vi "AutoFocus.vi"(0 "Function":T23, 1 "Set Inverse Matrix":T4, 5 "Displacement":dbl(slide) scale=1.0..1000.0, 7 "Matching Criteria":T7={"Minimum Score"=700.0, "Color Score Weight"=700.0, "Minimum Contrast"=50, "Match Mode"=0, "Match Feature Mode"=0, "Subpixel Accuracy"=TRUE, "Color Sensitivity"=1, "Search Strategy"=1} {"Match Mode" items=["Shift Invariant", "Rotation Invariant"]; "Match Feature Mode" items=["Color and Shape", "Color", "Shape"]; "Color Sensitivity" items=["Low Sensitivity", "Medium Sensitivity", "High Sensitivity"]; "Search Strategy" items=["Conservative", "Balance", "Aggressive", "Very Aggressive"]}, 9 "Z Scan Parameters":T3={"Z Range"=1380.0, "Resolution"=5000.0, "Initial Direction"=enum."Up", "Focus Threshold"=0.1, "Ascent Constant"=0.1} {"Focus Threshold" min=0.0 max=1000.0 step=1.0 format="%#_2f"; "Ascent Constant" min=0.0 max=1000.0 step=1.0 format="%#_2f"; "Resolution" min=0.0 max=1.0 step=0.01 format="%_2g"; "Z Range" format="%_3g"}, 11 "error in (no error)":errorcluster, 12 "Refnums":T21, 13 "Notifiers":T8, 14 "Message Queues out":T6) -> (4 "Target Found?":bool, 6 "Transformation Matrix":T4, 8 "Target Data":T5, 15 "error out":errorcluster)   [LabVIEW 2014]
uses:
  AutoFocus Functions.ctl
  AutoFocus Refnums.ctl
  support/Instrument Status.ctl
  ZScan.ctl
  <vilib>/Analysis/Matrix/Datatypes/RealMatrix.ctl
  Target Refnums.ctl
  support/Notifiers/Notifiers.ctl
  support/Message Handler Loop Notifiers.ctl
  Parameter Analyzer/Parameter Analyzer Notifiers.ctl
  Switching Matrix/Switching Matrix Notifiers.ctl
  Stress Control/StressControl Notifiers.ctl
  Spectrometer/Spectrometer Notifiers.ctl
  Switches and Mirrors/SwitchesMirrors Notifiers.ctl
  Camera/Camera Notifiers.ctl
  XYZ Stage/XYZ Notifications.ctl
  Autofocus Notifiers.ctl
  Measurements/Optoelectronic Measurement/Optoelectronic Notifiers.ctl
  Measurements/Save Data/SaveData Notifiers.ctl
  Measurements/Instrument Sequence/Instrument Sequence Notifiers.ctl
  support/Message Queue/All Message Queues.ctl
  support/Message Queue/Message Cluster.ctl
  support/Instrument Status State.ctl
  Target Functions.ctl
  <vilib>/Analysis/baseanly.llb/Matrix Type of Inverse Matrix.ctl
  XYZ Stage/XYZ Config.ctl
  XYZ Stage/XYZ Connection Settings.ctl
  XYZ Stage/XYZ Stage Control.ctl
  XYZ Stage/XYZ Coordinate Control.ctl
  <vilib>/Analysis/baseanly.llb/A x Vector.vi
  <vilib>/Analysis/baseanly.llb/Real Inverse Matrix.vi
  support/Message Queue/Message Queue.lvlib
  <vilib>/Analysis/NI_AALBase.lvlib
  <vilib>/Analysis/Matrix/NI_Matrix.lvlib
panel:
  out "Edge Detection Array":T1
  out "Instrument Status":T2
  out "Matching Curves":cluster{dbl[], sgl[]}[](graph)
  # "LICENSED MATERIALS – PROPERTY OF IBM\nCopyright IBM Corp. 2016,\nALL RIGHTS RESERVED"
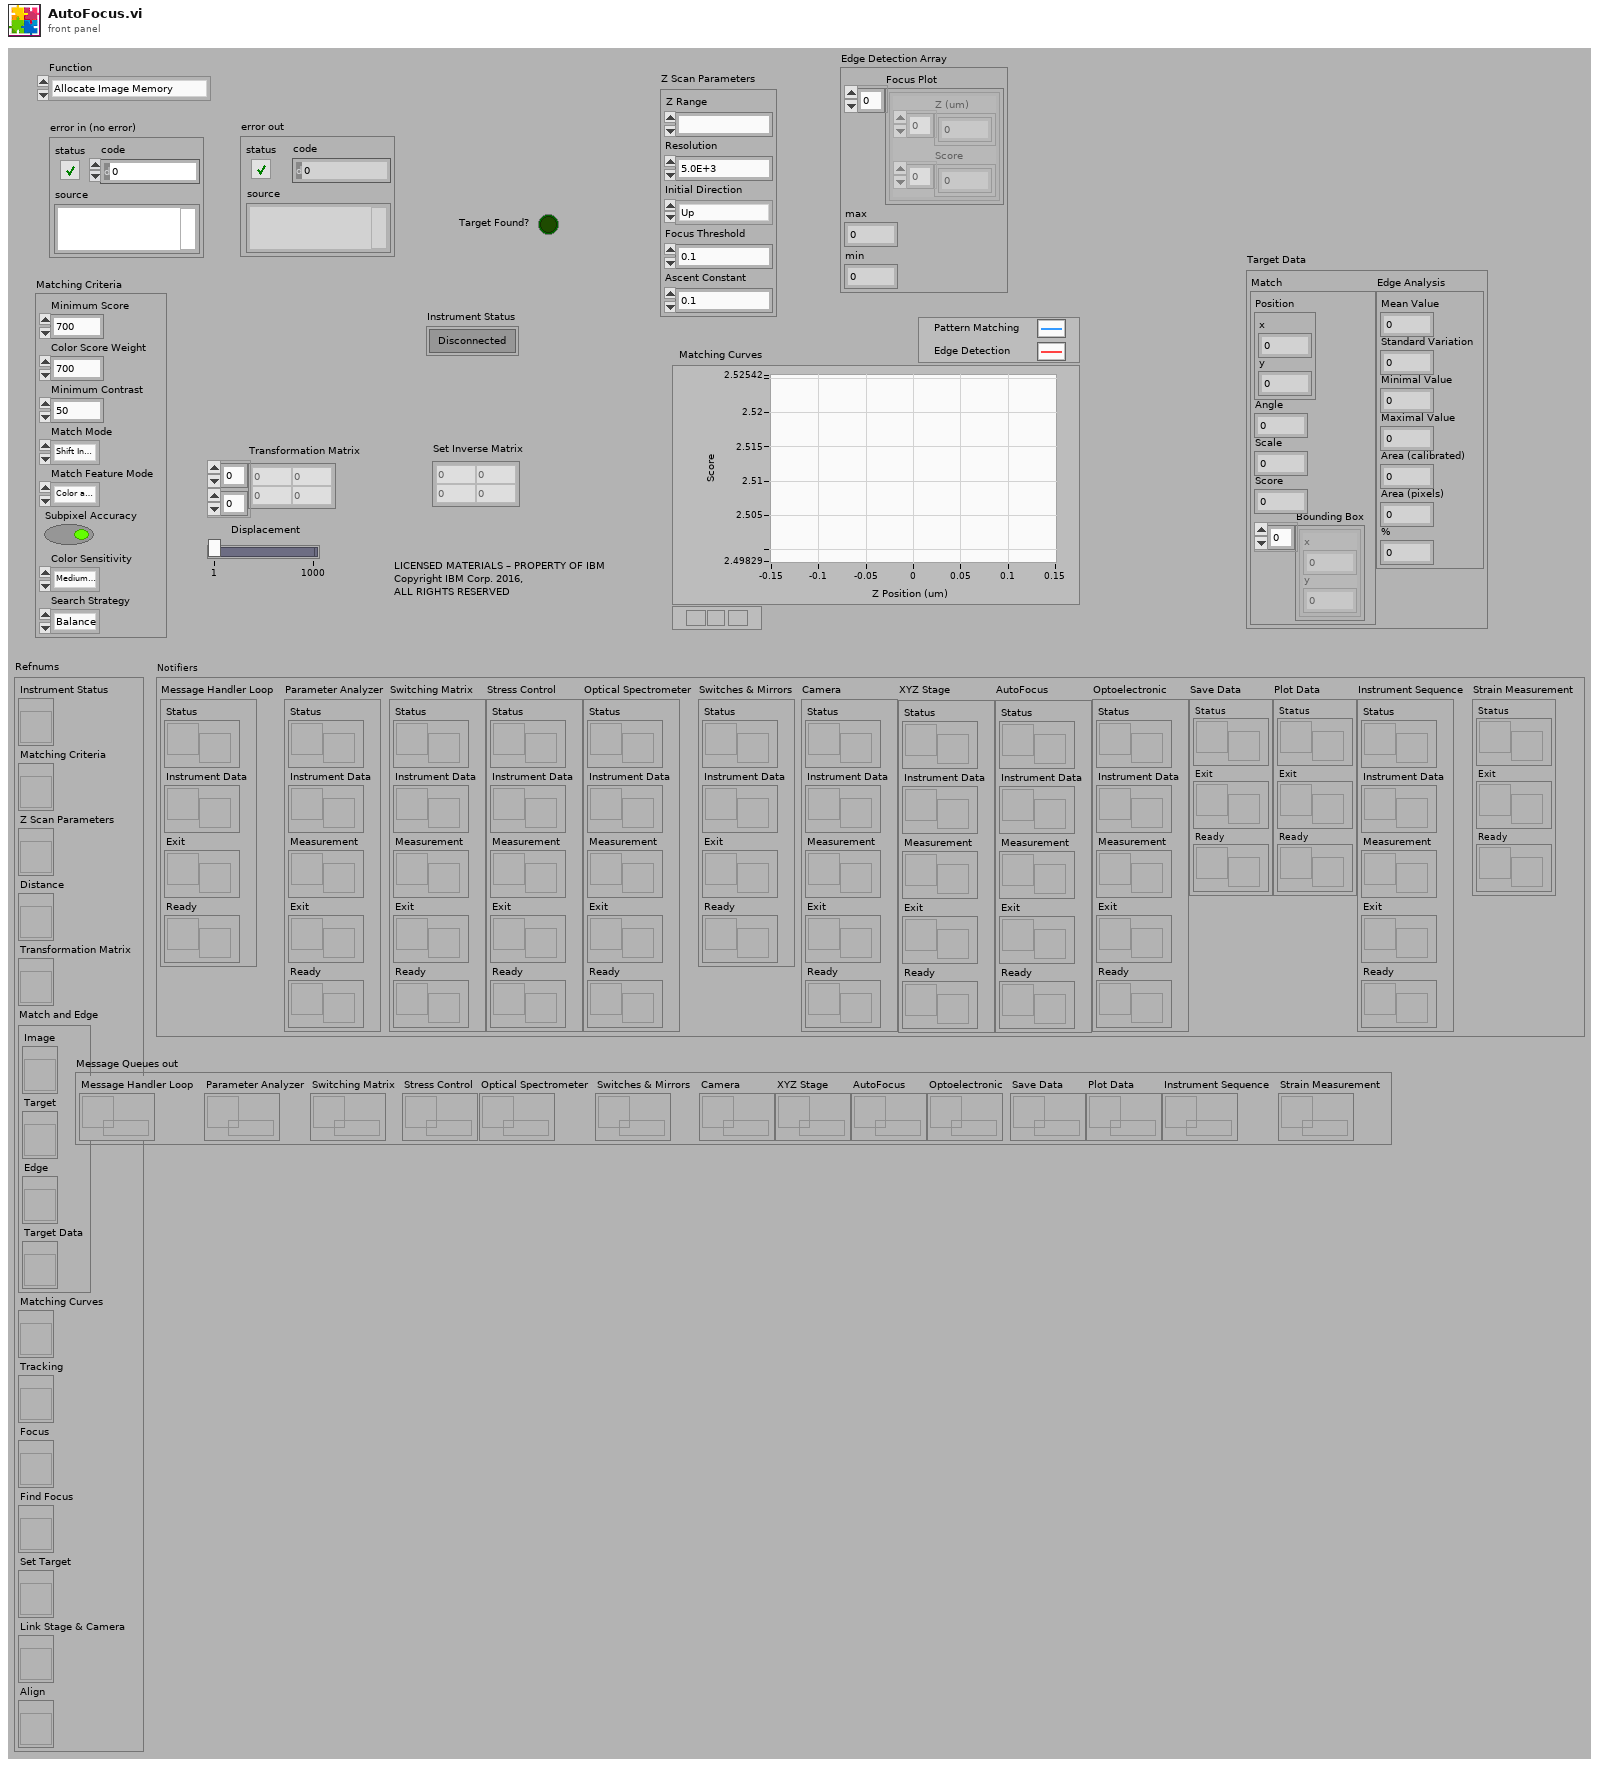
[diagram p1: front panel]
types:
  T1 = cluster{"Focus Plot":cluster{"Z (um)":dbl[], "Score":sgl[]}[], "max":sgl, "min":sgl}
  T2 = typedef "Instrument Status.ctl" = bool
  T3 = typedef "ZScan.ctl" = cluster{"Z Range":ext, "Resolution":dbl, "Initial Direction":enum16{"Up", "Down"}, "Focus Threshold":dbl, "Ascent Constant":dbl}
  T4 = typedef "NI_Matrix.lvlib/RealMatrix.ctl" = dbl[][]
  T5 = cluster{"Match":cluster{"Position":cluster{"x":sgl, "y":sgl}, "Angle":sgl, "Scale":sgl, "Score":sgl, "Bounding Box":cluster{"x":sgl, "y":sgl}[]}, "Edge Analysis":cluster{"Mean Value":sgl, "Standard Variation":sgl, "Minimal Value":sgl, "Maximal Value":sgl, "Area (calibrated)":sgl, "Area (pixels)":i32, "%":sgl}}
  T6 = typedef "Message Queue.lvlib/All Message Queues.ctl" = cluster{"Message Handler Loop":refnum<queue>, "Parameter Analyzer":refnum<queue>, "Switching Matrix":refnum<queue>, "Stress Control":refnum<queue>, "Optical Spectrometer":refnum<queue>, "Switches & Mirrors":refnum<queue>, "Camera":refnum<queue>, "XYZ Stage":refnum<queue>, "AutoFocus":refnum<queue>, "Optoelectronic":refnum<queue>, "Save Data":refnum<queue>, "Plot Data":refnum<queue>, "Instrument Sequence":refnum<queue>, "Strain Measurement":refnum<queue>}
  T7 = cluster{"Minimum Score":sgl, "Color Score Weight":sgl, "Minimum Contrast":i32, "Match Mode":u32, "Match Feature Mode":u32, "Subpixel Accuracy":bool, "Color Sensitivity":u32, "Search Strategy":u32}
  T8 = typedef "Notifiers.ctl" = cluster{"Message Handler Loop":T9, "Parameter Analyzer":T10, "Switching Matrix":T11, "Stress Control":T12, "Optical Spectrometer":T13, "Switches & Mirrors":T14, "Camera":T15, "XYZ Stage":T16, "AutoFocus":T17, "Optoelectronic":T18, "Save Data":T19, "Plot Data":T19, "Instrument Sequence":T20, "Strain Measurement":cluster{"Status":refnum<notifier>, "Exit":refnum<notifier>, "Ready":refnum<notifier>}}
  T9 = typedef "Message Handler Loop Notifiers.ctl" = cluster{"Status":refnum<notifier>, "Instrument Data":refnum<notifier>, "Exit":refnum<notifier>, "Ready":refnum<notifier>}
  T10 = typedef "Parameter Analyzer Notifiers.ctl" = cluster{"Status":refnum<notifier>, "Instrument Data":refnum<notifier>, "Measurement":refnum<notifier>, "Exit":refnum<notifier>, "Ready":refnum<notifier>}
  T11 = typedef "Switching Matrix Notifiers.ctl" = cluster{"Status":refnum<notifier>, "Instrument Data":refnum<notifier>, "Measurement":refnum<notifier>, "Exit":refnum<notifier>, "Ready":refnum<notifier>}
  T12 = typedef "StressControl Notifiers.ctl" = cluster{"Status":refnum<notifier>, "Instrument Data":refnum<notifier>, "Measurement":refnum<notifier>, "Exit":refnum<notifier>, "Ready":refnum<notifier>}
  T13 = typedef "Spectrometer Notifiers.ctl" = cluster{"Status":refnum<notifier>, "Instrument Data":refnum<notifier>, "Measurement":refnum<notifier>, "Exit":refnum<notifier>, "Ready":refnum<notifier>}
  T14 = typedef "SwitchesMirrors Notifiers.ctl" = cluster{"Status":refnum<notifier>, "Instrument Data":refnum<notifier>, "Exit":refnum<notifier>, "Ready":refnum<notifier>}
  T15 = typedef "Camera Notifiers.ctl" = cluster{"Status":refnum<notifier>, "Instrument Data":refnum<notifier>, "Measurement":refnum<notifier>, "Exit":refnum<notifier>, "Ready":refnum<notifier>}
  T16 = typedef "XYZ Notifications.ctl" = cluster{"Status":refnum<notifier>, "Instrument Data":refnum<notifier>, "Measurement":refnum<notifier>, "Exit":refnum<notifier>, "Ready":refnum<notifier>}
  T17 = typedef "Autofocus Notifiers.ctl" = cluster{"Status":refnum<notifier>, "Instrument Data":refnum<notifier>, "Measurement":refnum<notifier>, "Exit":refnum<notifier>, "Ready":refnum<notifier>}
  T18 = typedef "Optoelectronic Notifiers.ctl" = cluster{"Status":refnum<notifier>, "Instrument Data":refnum<notifier>, "Measurement":refnum<notifier>, "Exit":refnum<notifier>, "Ready":refnum<notifier>}
  T19 = typedef "SaveData Notifiers.ctl" = cluster{"Status":refnum<notifier>, "Exit":refnum<notifier>, "Ready":refnum<notifier>}
  T20 = typedef "Instrument Sequence Notifiers.ctl" = cluster{"Status":refnum<notifier>, "Instrument Data":refnum<notifier>, "Measurement":refnum<notifier>, "Exit":refnum<notifier>, "Ready":refnum<notifier>}
  T21 = typedef "AutoFocus Refnums.ctl" = cluster{"Instrument Status":refnum<vi>, "Matching Criteria":refnum<vi>, "Z Scan Parameters":refnum<vi>, "Distance":refnum<vi>, "Transformation Matrix":refnum<vi>, "Match and Edge":T22, "Matching Curves":refnum<vi>, "Tracking":refnum<vi>, "Focus":refnum<vi>, "Find Focus":refnum<vi>, "Set Target":refnum<vi>, "Link Stage & Camera":refnum<vi>, "Align":refnum<vi>}
  T22 = typedef "Target Refnums.ctl" = cluster{"Image":refnum<vi>, "Target":refnum<vi>, "Edge":refnum<vi>, "Target Data":refnum<vi>}
  T23 = typedef "AutoFocus Functions.ctl" = enum16{"Allocate Image Memory", "Free Image Memory", "Grab Image", "Get ROI", "Set ROI", "Set Match Criteria", "Set Target", "Link Stage & Camera", "Set Transformation Matrix", "Find Target", "Align", "Find Focus", "Focus (Gradient)", "Focus (Threshold)", "Focus (Turning Points)", "Update Refnums"}
  T24 = typedef "Instrument Status State.ctl" = enum16{"Unknown", "Idle", "Standby", "Configuring", "Measuring", "Moving", "Disconnected"}
  T25 = typedef "Image Type" = u32
  T26 = cluster{"Border Size":i32, "Image Name":string, "Image Type":T25}[]
  T27 = typedef "Target Functions.ctl" = enum16{"Setup Match Criteria", "Set Target", "Find Target"}
  T28 = typedef "NI_AALBase.lvlib/Matrix Type of Inverse Matrix.ctl" = enum32{"General", "Positive Definite", "Lower Triangular", "Upper Triangular"}
  T29 = typedef "XYZ Config.ctl" = cluster{"Connection Settings":T30, "Manual Control":T31, "Coordinate Control":T32}
  T30 = typedef "XYZ Connection Settings.ctl" = cluster{"Tango VISA":refnum<visa-resource-name>, "Baudrate":i32, "Show Protocol?":bool}
  T31 = typedef "XYZ Stage Control.ctl" = cluster{"North":bool, "South":bool, "West":bool, "East":bool, "Up":bool, "Down":bool, "Stop":bool, "XY Step":dbl, "Z step":dbl}
  T32 = typedef "XYZ Coordinate Control.ctl" = cluster{"Motion Mode":enum16{"Absolute", "Relative"}, "Destination [mm]":dbl[]}
  T33 = typedef "IMAQ Image.ctl" = refnum<image>
  T34 = cluster{"Global Rectangle":i32[], "Contours":cluster{"Contour Type":u32, "ROI Type":u32, "Points":i32[]}[]}
  T35 = cluster{"Registers Filled?":bool, "Negative Edge Slope?":bool, "Negative Z Slope?":bool, "Focus at Edge?":bool}
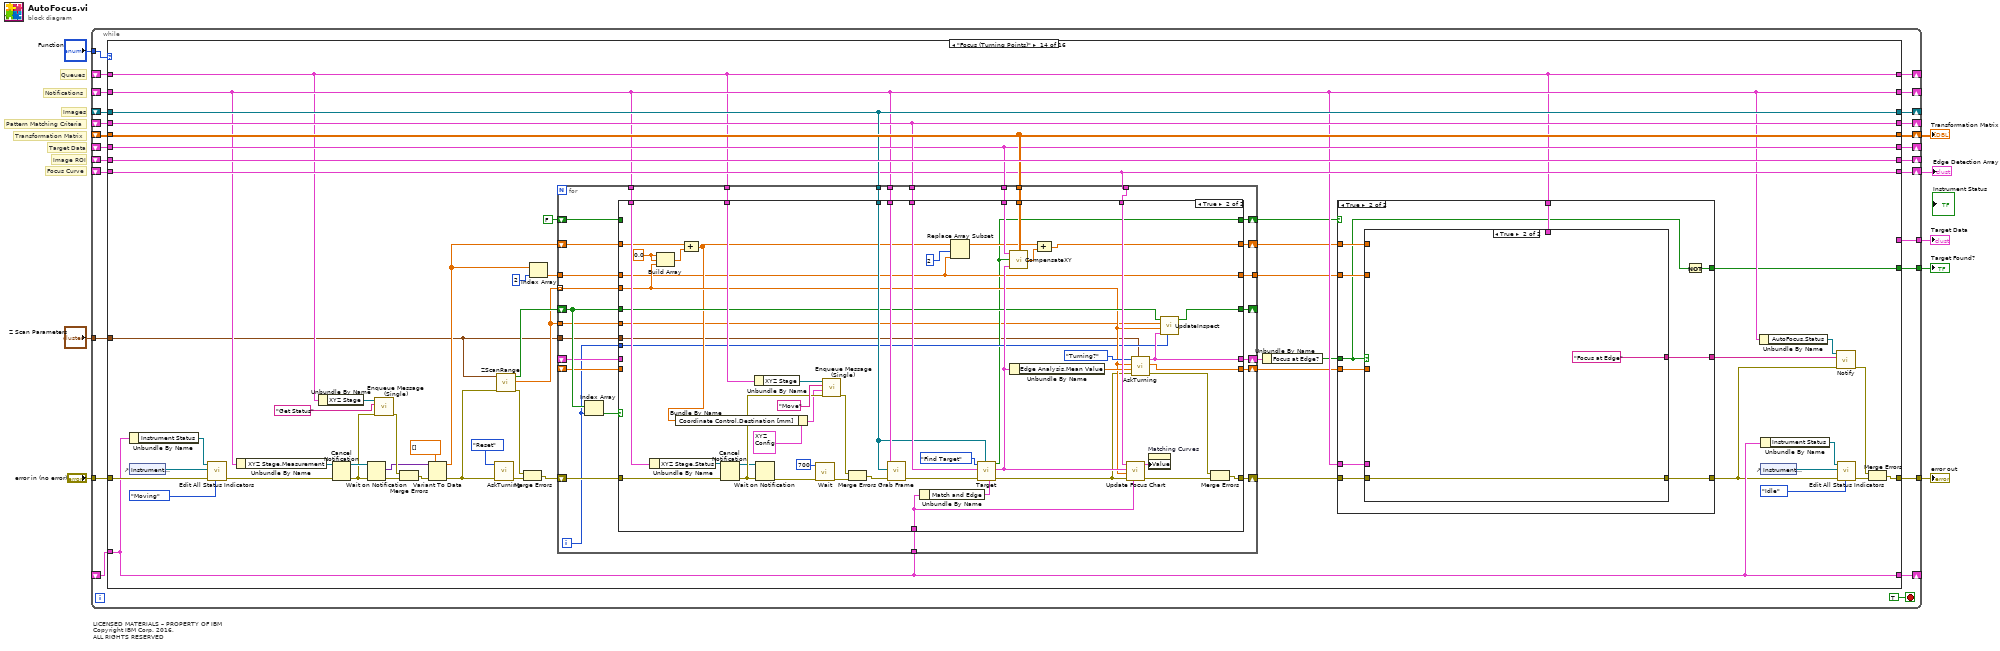
[diagram p0: block diagram]
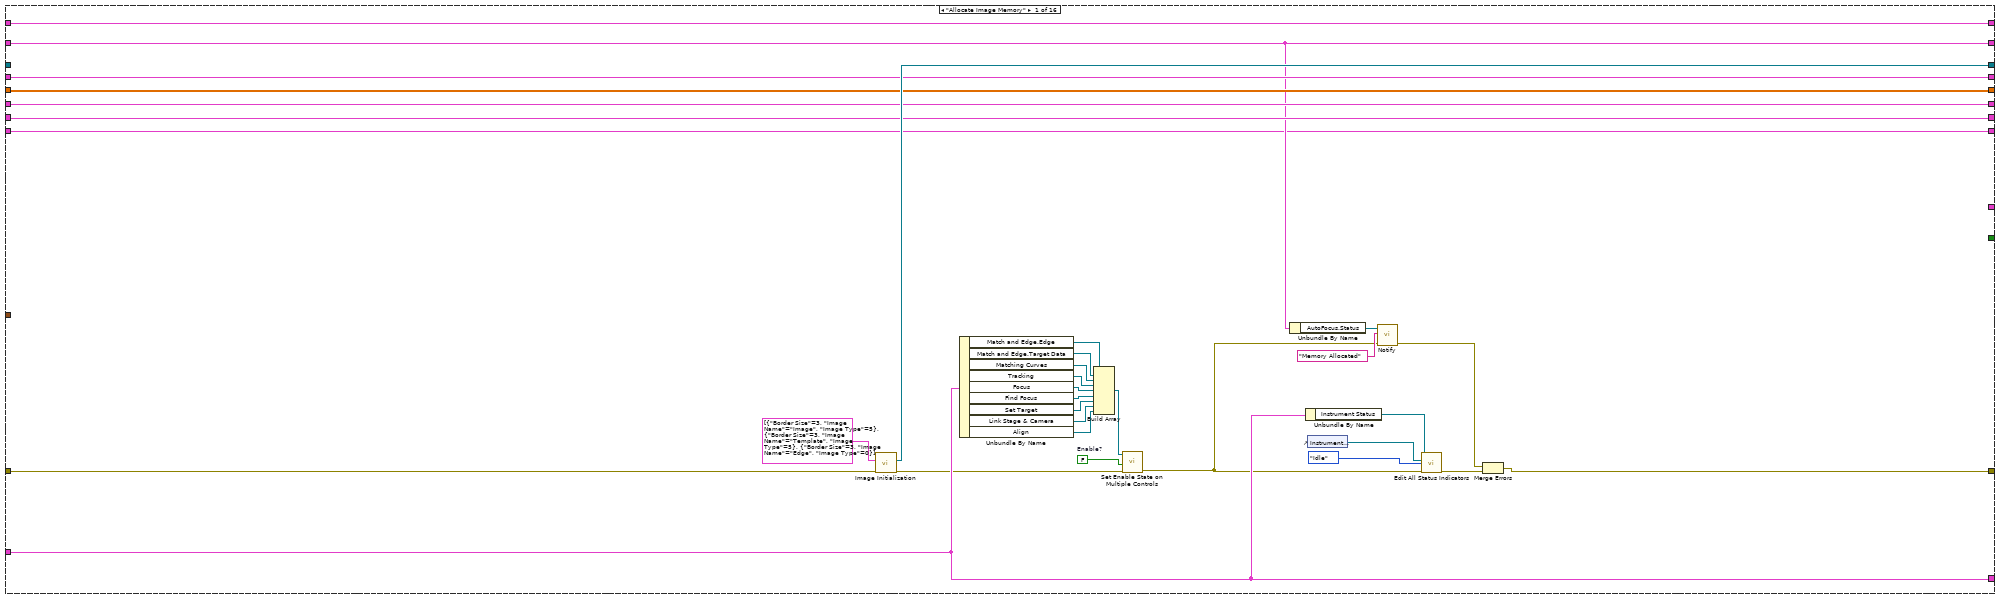
[diagram p2: hidden frame]
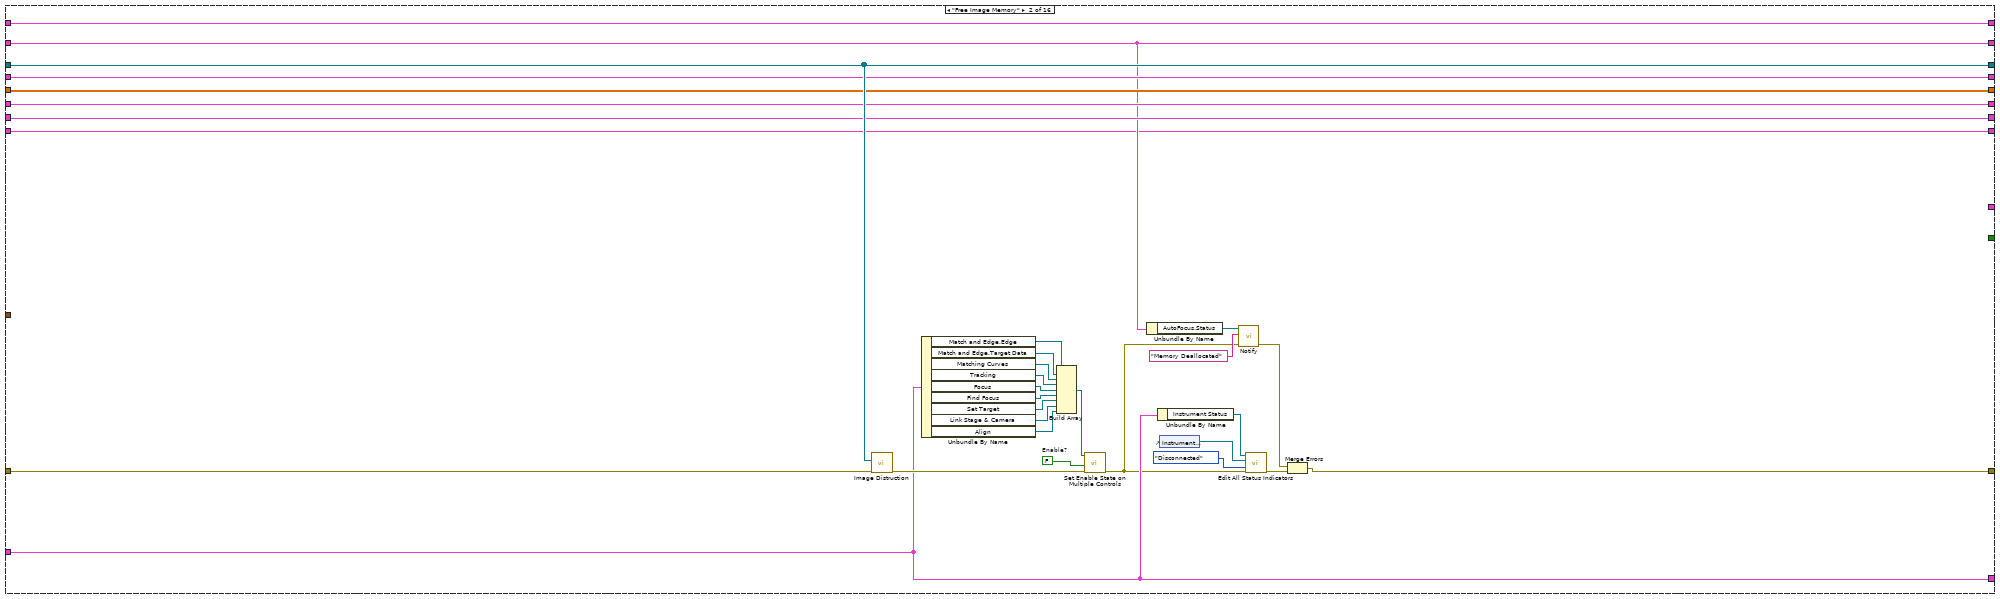
[diagram p3: hidden frame]
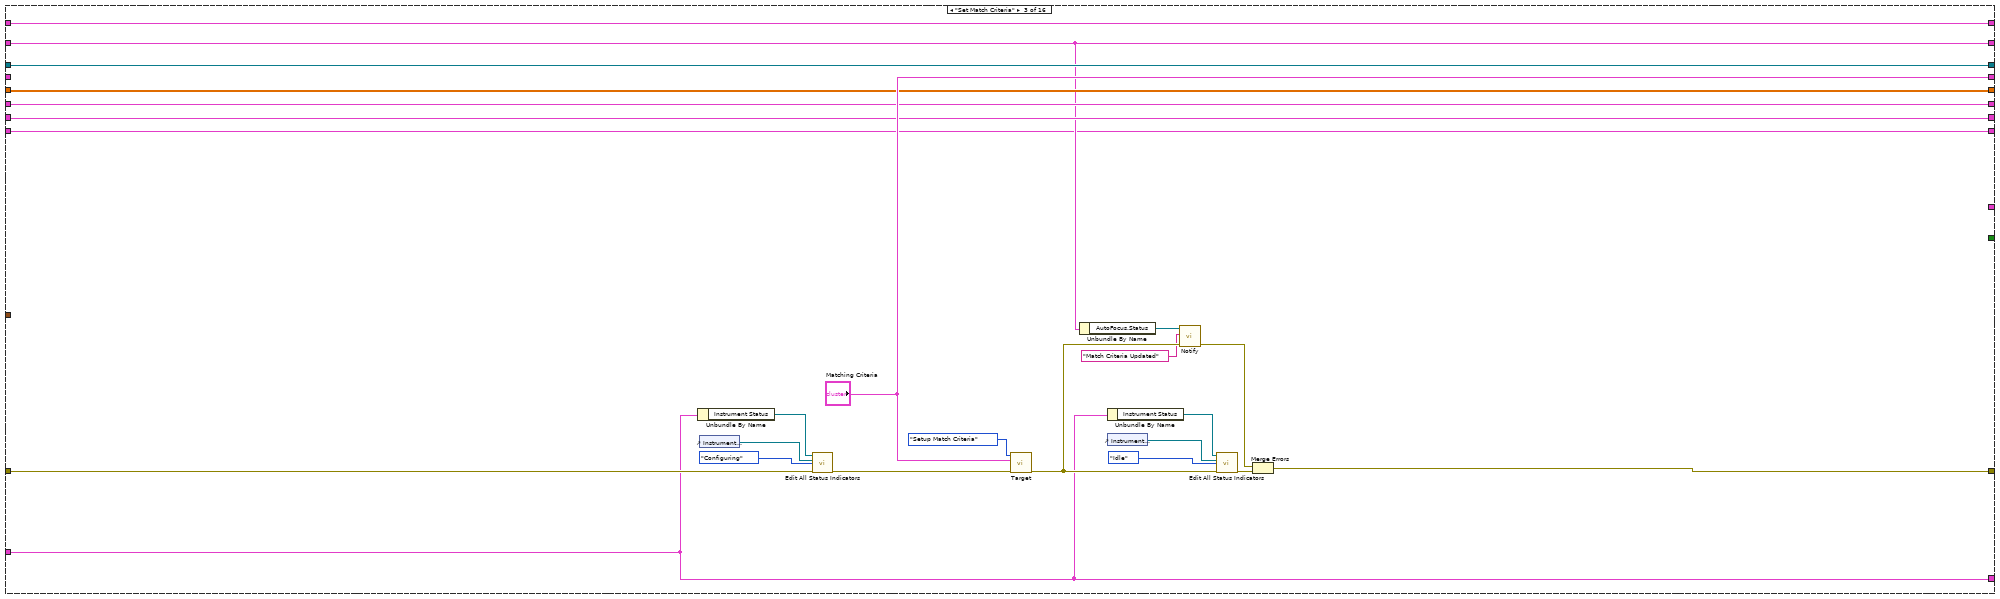
[diagram p4: hidden frame]
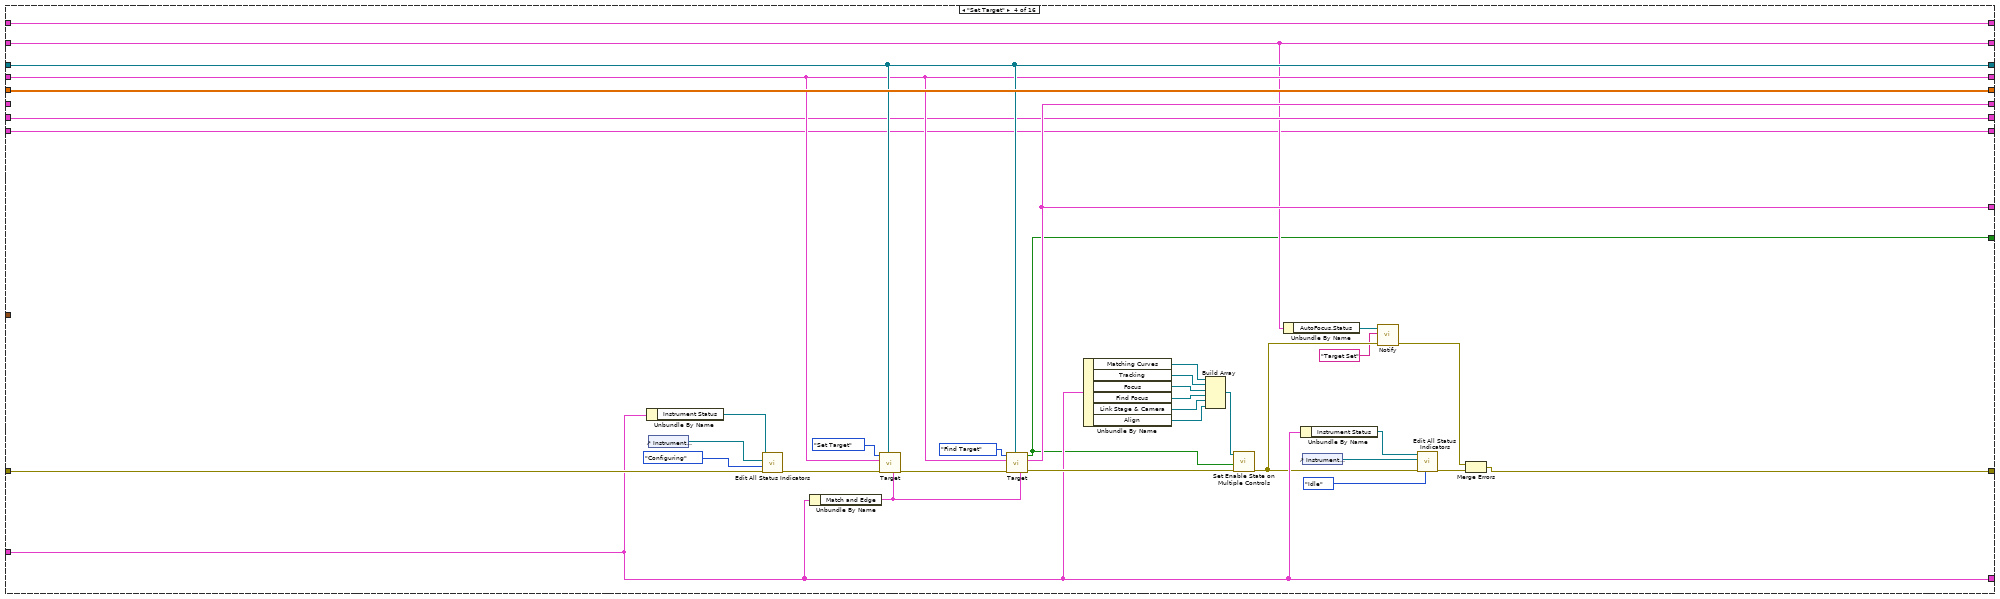
[diagram p5: hidden frame]
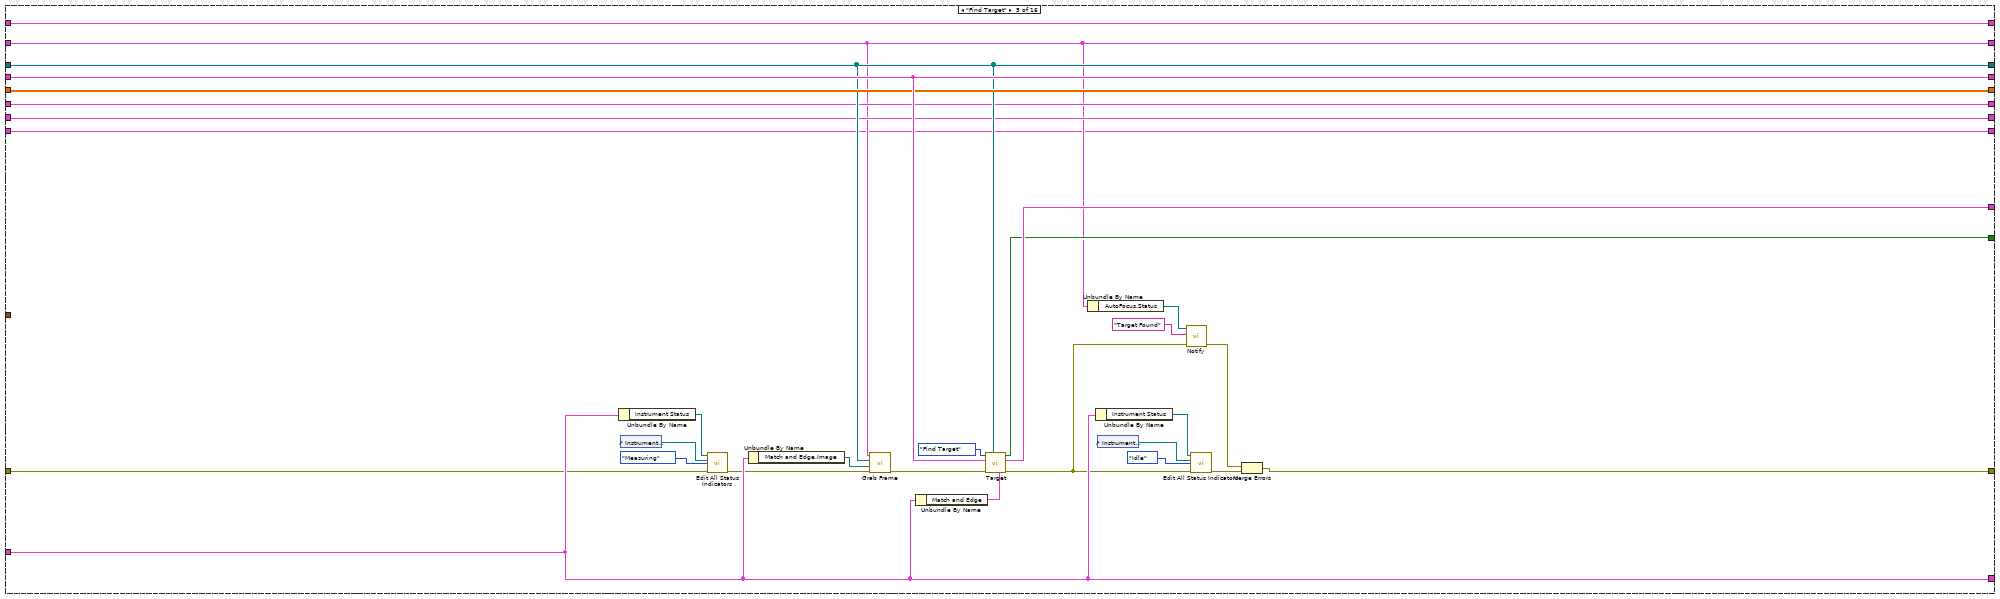
[diagram p6: hidden frame]
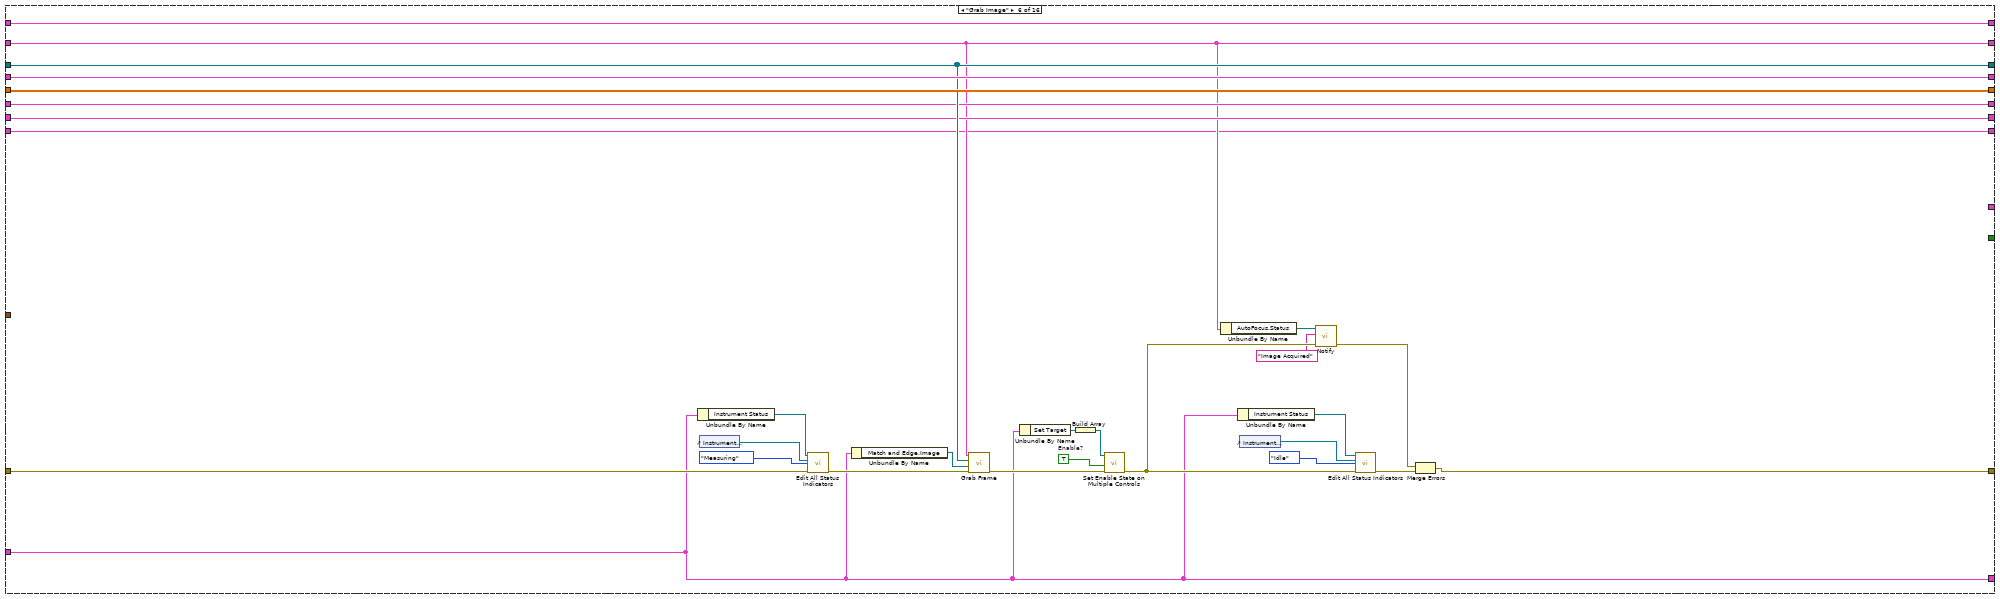
[diagram p7: hidden frame]
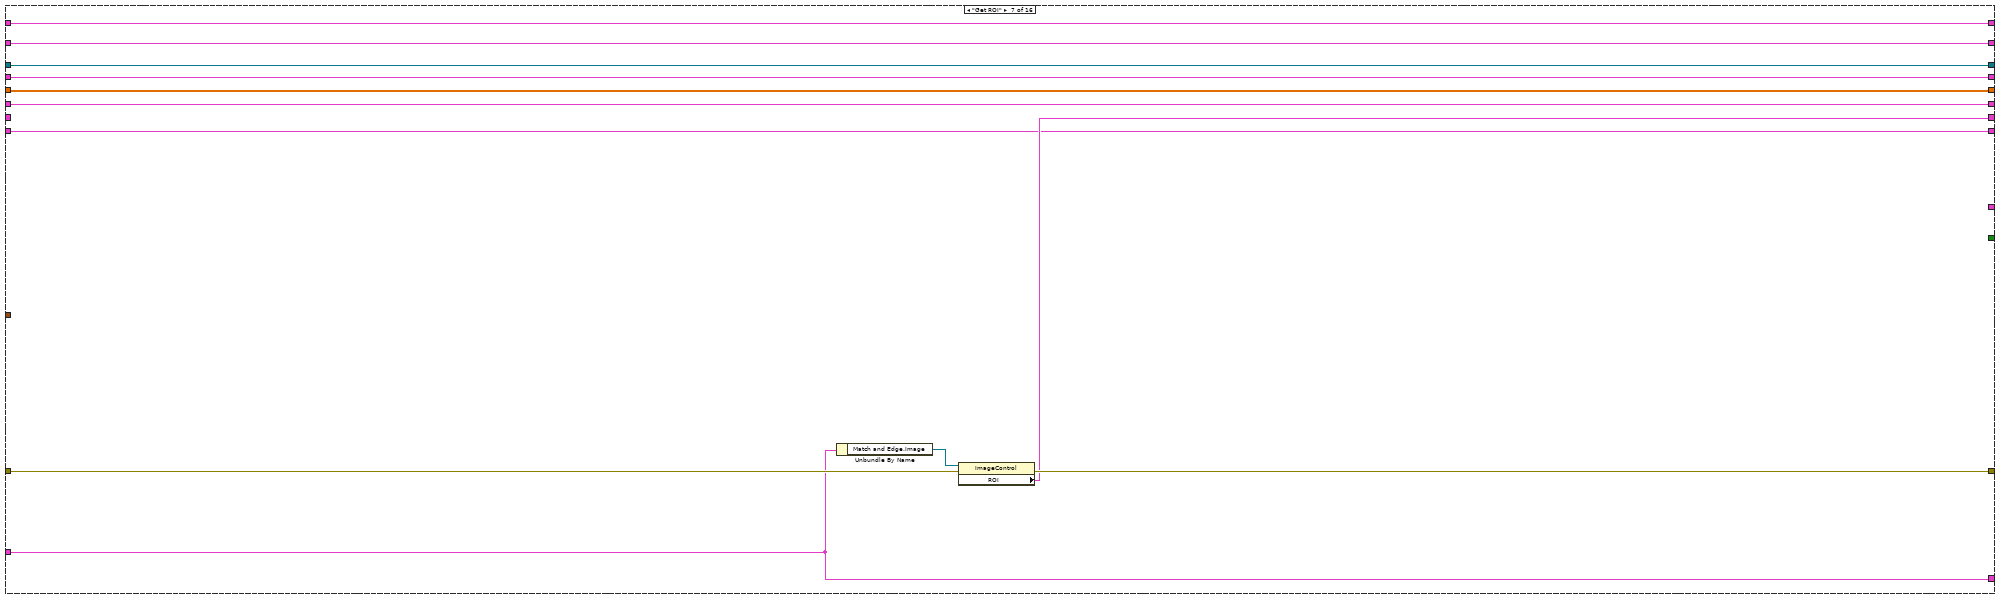
[diagram p8: hidden frame]
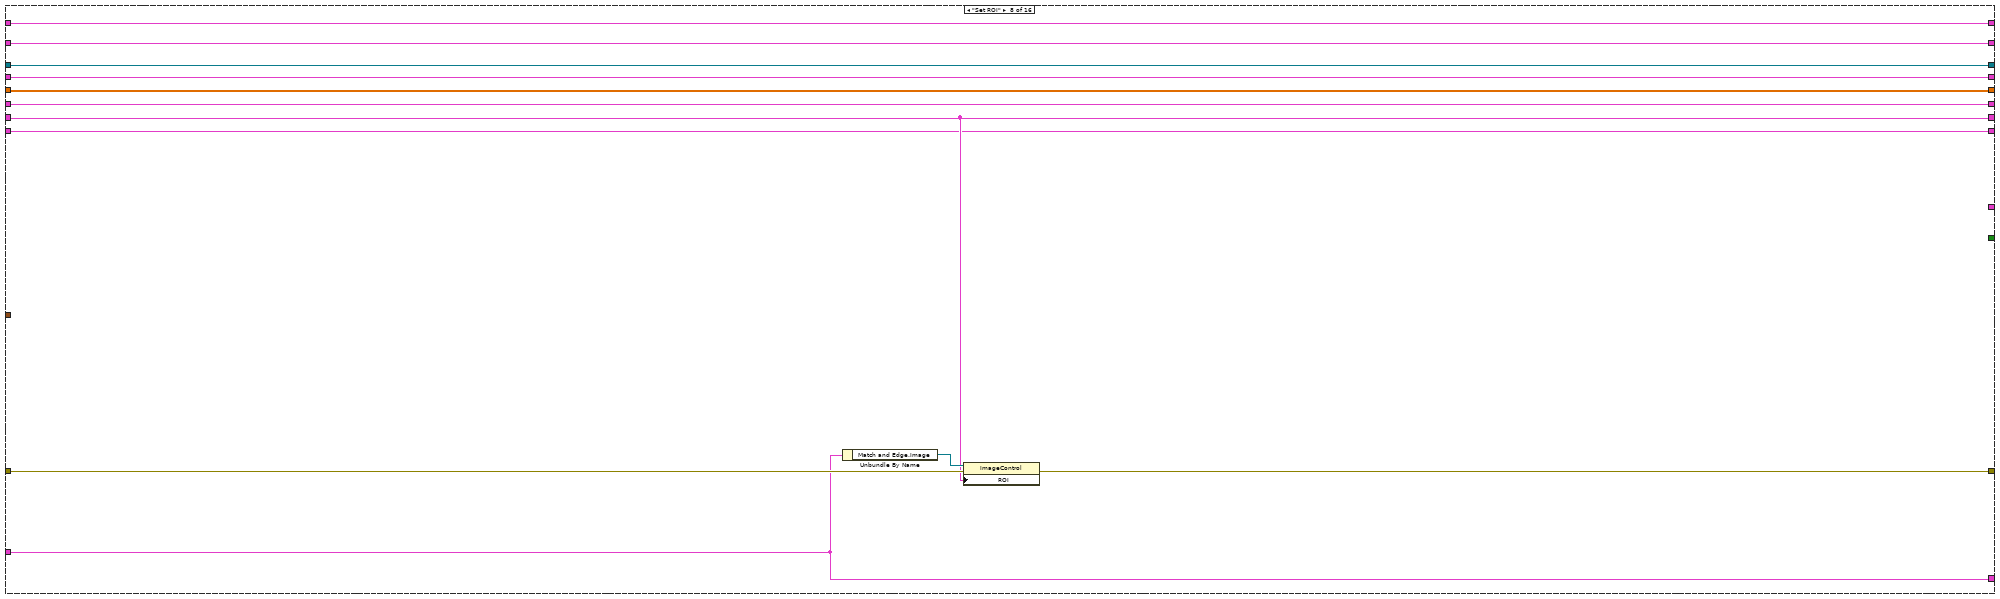
[diagram p9: hidden frame]
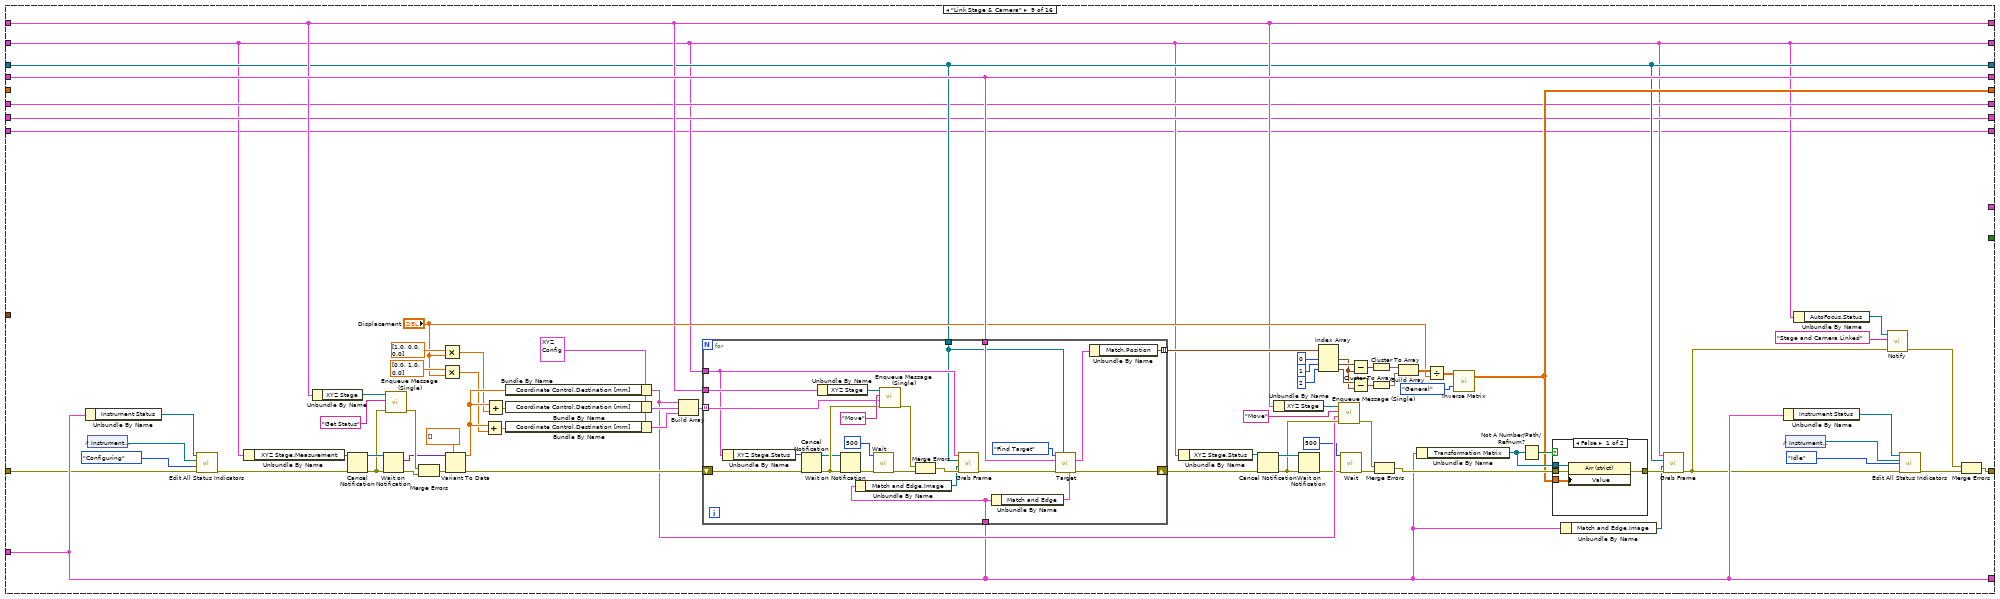
[diagram p10: hidden frame]
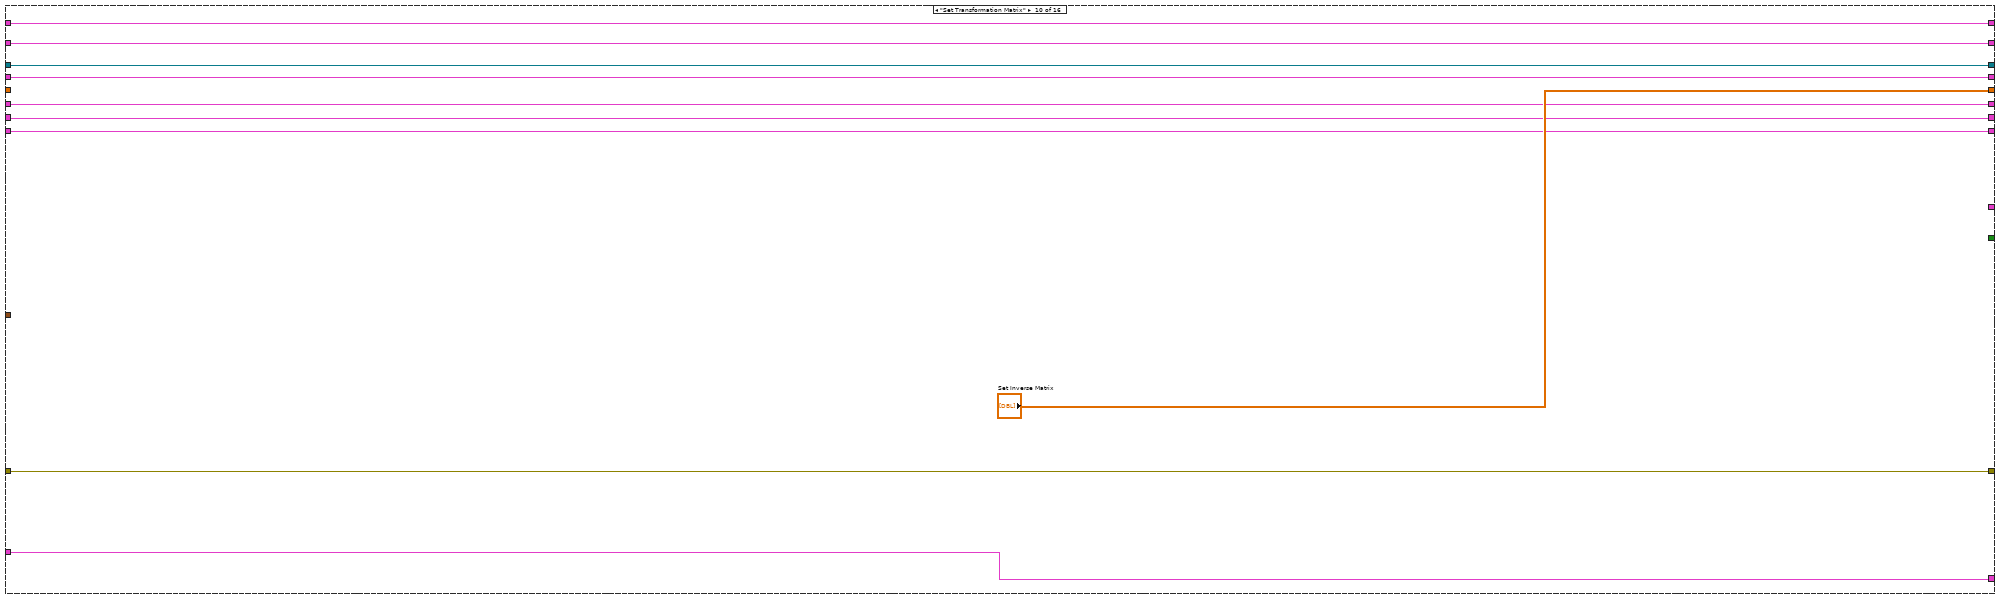
[diagram p12: hidden frame]
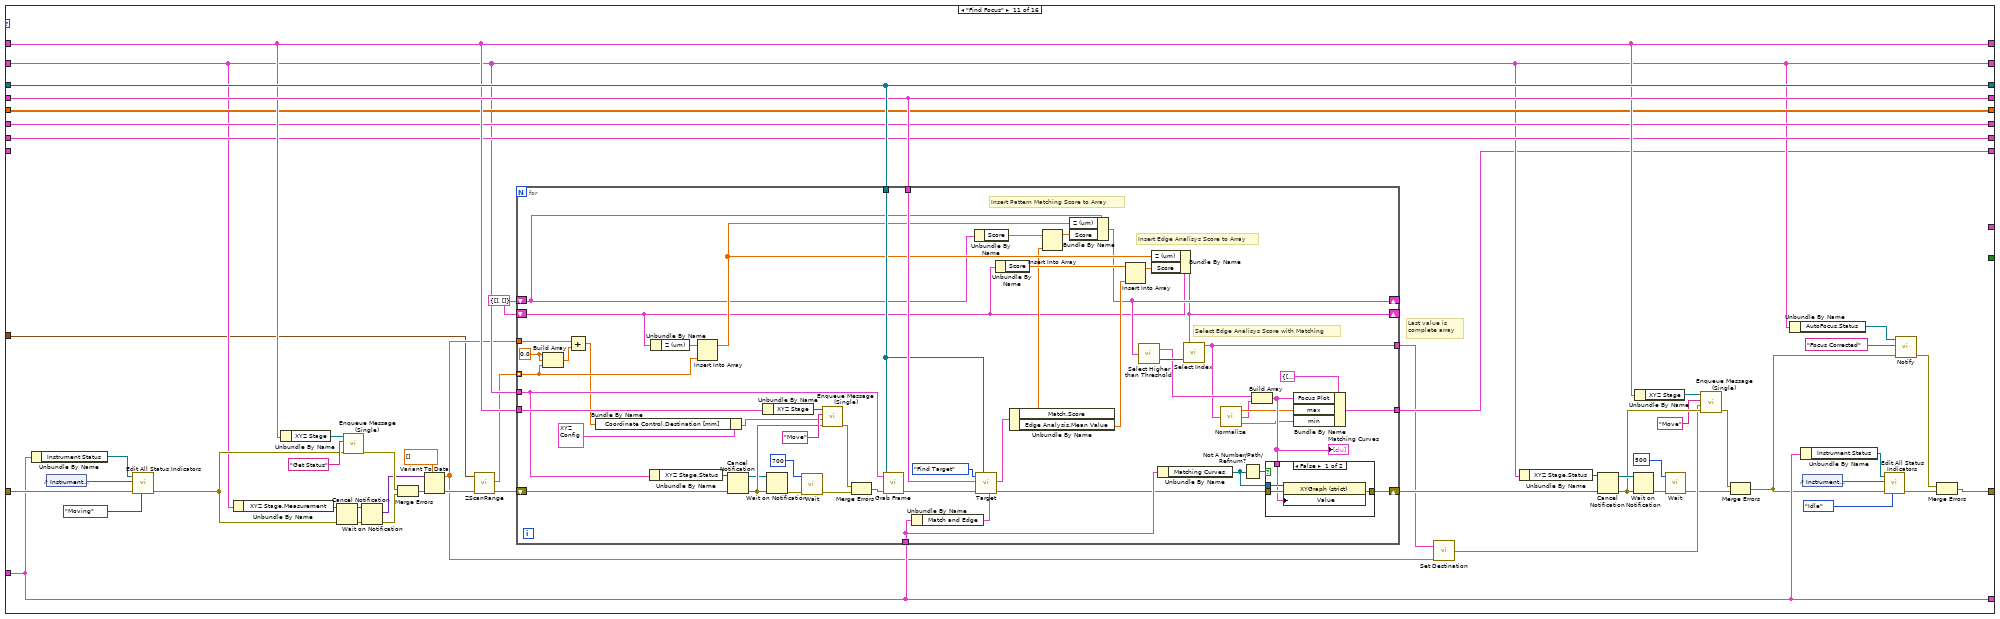
[diagram p13: hidden frame]
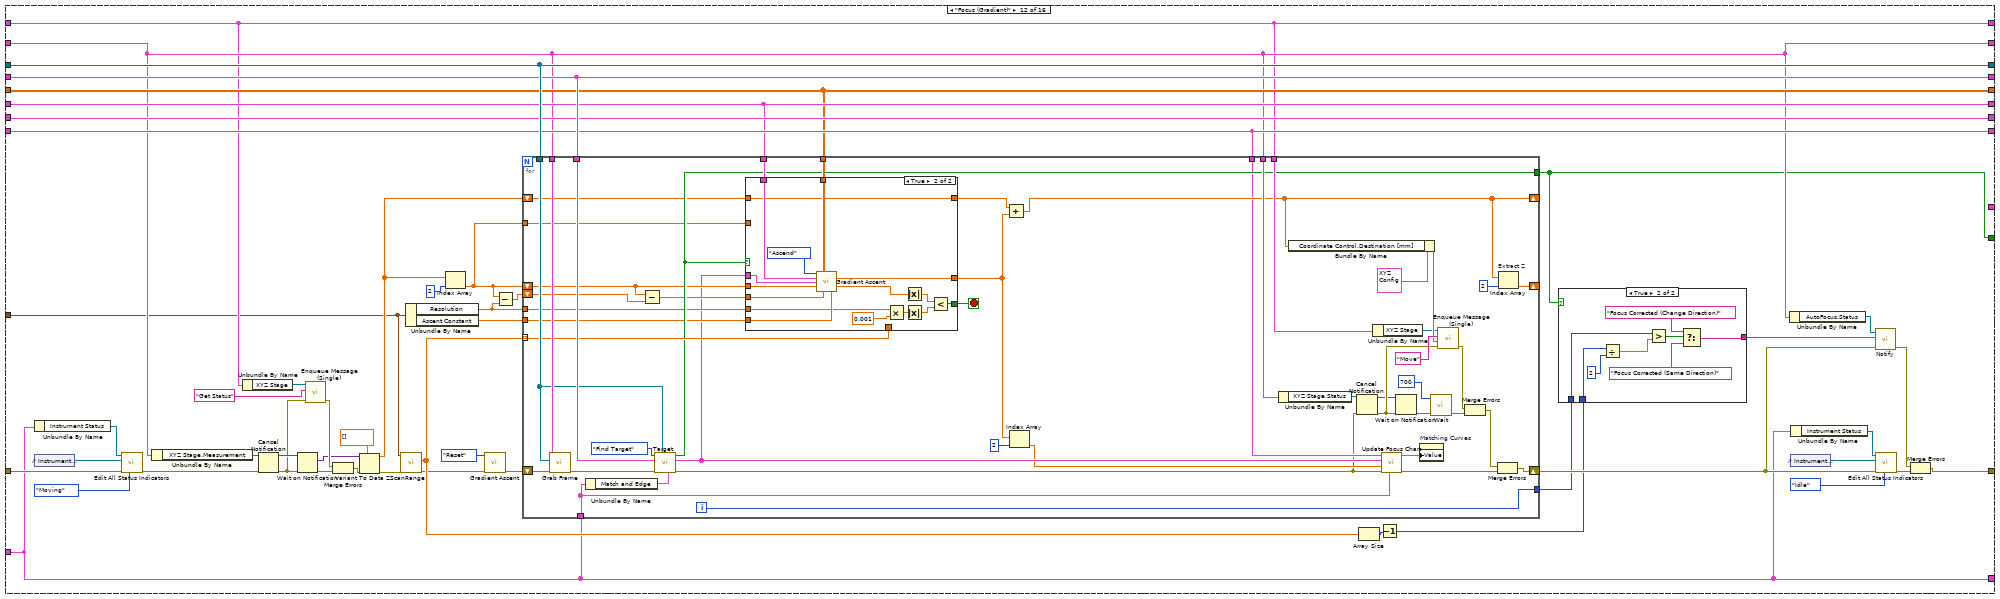
[diagram p15: hidden frame]
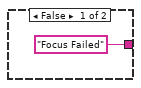
[diagram p16: hidden frame]
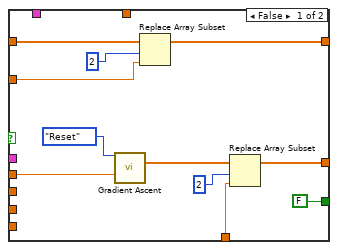
[diagram p17: hidden frame]
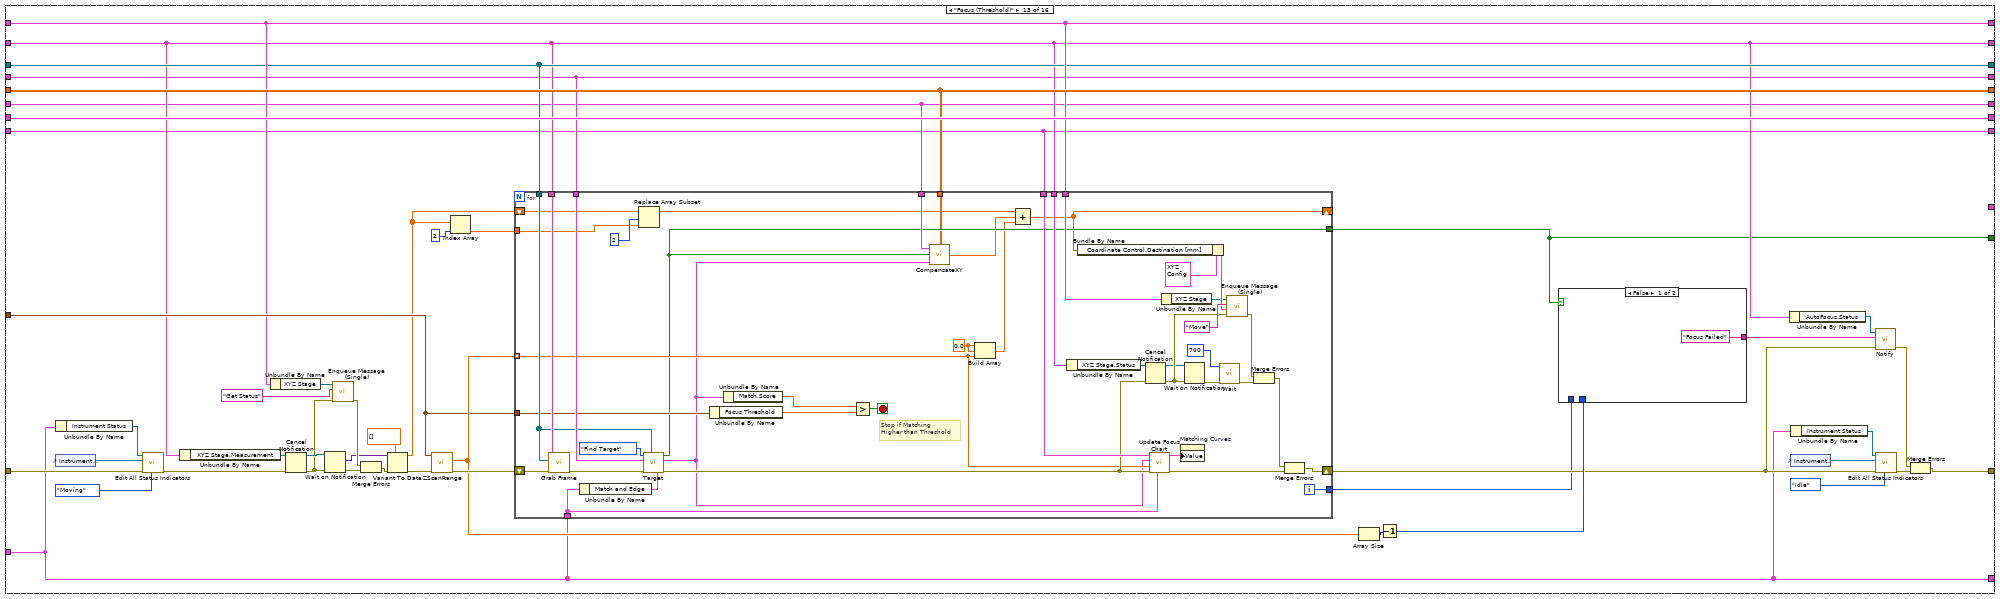
[diagram p18: hidden frame]
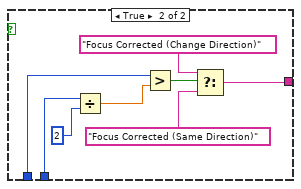
[diagram p19: hidden frame]
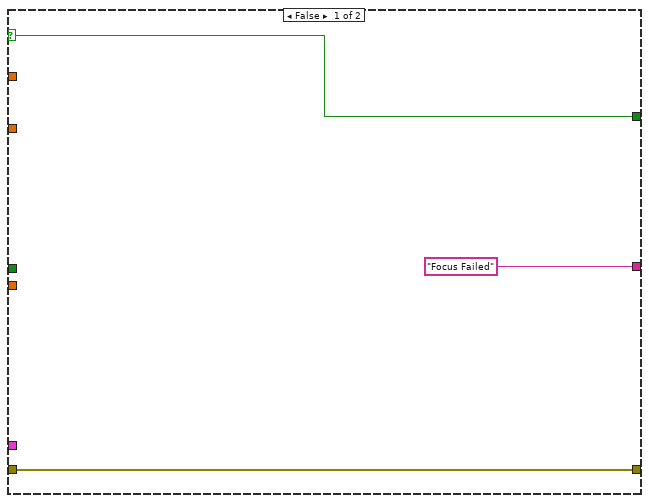
[diagram p20: hidden frame]
diagram:
  # "LICENSED MATERIALS – PROPERTY OF IBM\nCopyright IBM Corp. 2016,\nALL RIGHTS RESERVED"
  # "Focus Curve"
  # "Image ROI"
  # "Target Data"
  # "Notifications"
  # "Queues"
  # "Transformation Matrix"
  # "Pattern Matching Criteria"
  # "Images"
  n1 = while {
    tunnel: "Function" -> [w33]
    tunnel: "error in (no error)" -> [w32]
    tunnel: [w31] -> w6
    shift-right: [w30] -> _
    shift-left: _ -> [w29]
    shift-right: [w27] -> _
    shift-left: _ -> [w26]
    shift-right: [w25] -> _
    shift-left: _ -> [w24]
    shift-right: [w23] -> _
    shift-left: _ -> [w22]
    shift-right: [w20] -> _
    shift-left: _ -> [w21]
    shift-right: [w19] -> w5
    shift-left: _ -> [w18]
    shift-right: [w17] -> _
    shift-left: _ -> [w16]
    tunnel: [w15] -> w4
    tunnel: [w14] -> w3
    shift-right: [w12] -> _
    shift-left: _ -> [w13]
    shift-right: [w11] -> w1
    shift-left: _ -> [w10]
    tunnel: "Z Scan Parameters" -> [w9]
    stop <- TRUE stop-if-true
    n2 = case shown="\"Focus (Turning Points)\"" w33 {
      tunnel: w32 -> [w64 w96 w108 w143 w168 w202 w218 w230 w252 w346 w375 w481 w618 w728 w884 w930]
      tunnel: [w54 w87 w109 w142 w172 w201 w217 w229 w250 w346 w372 w494 w623 w731 w886 w929] -> w31
      tunnel: [w63 w95 w120 w151 w180 w210 w221 w233 w261 w352 w403 w509 w601 w716 w891 w941] -> w30
      tunnel: w29 -> [_ w95 w120 w151 w180 w210 w221 w233 w261 w352 w403 w509 w601 w716 w891 w941]
      tunnel: [w56 w75 w106 w131 w171 w194 w216 w228 w253 w348 w370 w478 w602 w717 w883 "Refnums"] -> w27
      tunnel: w26 -> [w56 w75 w106 w131 w171 w194 w216 w228 w253 w348 w370 w478 w602 w717 w883 _]
      tunnel: [w62 w94 "Matching Criteria" w150 w183 w213 w225 w237 w313 w351 w402 w508 w599 w715 w898 w939] -> w25
      tunnel: w24 -> [w62 w94 _ w150 w183 w213 w225 w237 w313 w351 w402 w508 w599 w715 w898 w939]
      tunnel: [w57 w86 w105 w141 w170 w200 w222 w234 w254 w350 w371 w486 w600 w702 w885 "Notifiers"] -> w23
      tunnel: w22 -> [w57 w86 w105 w141 w170 w200 w222 w234 w254 w350 w371 w486 w600 w702 w885 _]
      tunnel: w21 -> [w61 w93 w117 w155 w182 w212 w224 w236 w269 w349 w391 w485 w603 w699 w896 _]
      tunnel: [w61 w93 w117 w155 w182 w212 w224 w236 w269 w349 w391 w485 w603 w699 w896 "Message Queues out"] -> w20
      tunnel: [w60 w92 w116 w154 w181 w211 w223 w235 w265 "Set Inverse Matrix" w390 w487 w604 w718 w892 w937] -> w19
      tunnel: w18 -> [w60 w92 w116 w154 w181 w211 w223 w235 _ _ w390 w487 w604 w718 w892 w937]
      tunnel: [w59 w91 w115 w148 w177 w208 w220 w232 w257 w345 w387 w491 w598 w714 w890 w936] -> w17
      tunnel: w16 -> [w59 w91 w115 _ w177 w208 w220 w232 w257 w345 w387 w491 w598 w714 w890 w936]
      tunnel: [_ _ _ w148 w176 _ _ _ _ _ _ _ _ _ w880 _] -> w15
      tunnel: [_ _ _ w130 w175 _ _ _ _ _ _ w472 w597 w693 w881 _] -> w14
      tunnel: w13 -> [w58 w90 w114 w147 w174 w207 _ w227 w256 w344 w376 w498 w627 w735 w888 w935]
      tunnel: [w58 w90 w114 w147 w174 w207 w215 w227 w256 w344 w376 w498 w627 w735 w888 w935] -> w12
      tunnel: [w41 w72 w104 w128 w167 w193 w214 w226 w249 w343 w366 w493 w594 w711 w882 w933] -> w11
      tunnel: w10 -> [w41 w72 w104 w128 w167 w193 w214 w226 w249 w343 _ w493 w594 w711 w882 w933]
      tunnel: w9 -> [_ _ _ _ _ _ _ _ _ _ w363 w469 w607 w692 _ _]
      frame "Allocate Image Memory" {
        w43 = FALSE  # Enable?
        n3 = call "Image Initialization.vi"("error in"=w64, "Image Definition"=T26 [{"Border Size"=3, "Image Name"="Image", "Image Type"=5}, {"Border Size"=3, "Image Name"="Template", "Image Type"=5}, {"Border Size"=3, "Image Name"="Edge", "Image Type"=0}]) -> ("error out"=w53:errorcluster, "Images"=w63:T33[])  [unwired: 1 in, 7 out]
        n4 = Unbundle By Name(w56) -> ("Match and Edge.Edge"=w42:refnum<vi>, "Match and Edge.Target Data"=w52:refnum<vi>, "Matching Curves"=w51:refnum<vi>, "Tracking"=w50:refnum<vi>, "Focus"=w49:refnum<vi>, "Find Focus"=w48:refnum<vi>, "Set Target"=w47:refnum<vi>, "Link Stage & Camera"=w46:refnum<vi>, "Align"=w45:refnum<vi>)
        n5 = Build Array(w42, w52, w51, w50, w49, w48, w47, w46, w45) -> (w44:refnum<vi>[])
        n6 = call "Set Enable State on Multiple Controls.vi"("error in (no error)"=w53, "Enable?"=w43, "Controls"=w44) -> ("error out"=w39:errorcluster)  [unwired: 8 in]
        n7 = Unbundle By Name(w57) -> ("AutoFocus.Status"=w38:refnum<notifier>)
        n8 = Unbundle By Name(w56) -> ("Instrument Status"=w36:refnum<vi>)
        n9 = control-ref of="Instrument Status"() -> (w35:refnum<vi>)
        n10 = call "Notify.vi"("error in (no error)"=w39, "String"="Memory Allocated", "Notifier in"=w38) -> ("error out"=w37:errorcluster)  [unwired: 8 in]
        n11 = call "Edit All Status Indicators.vi"("Instrument Status Ouside"=w36, "Instrument Status Inside"=w35, "Error In"=w39, "State"=Instrument_Status_State."Idle") -> ("Error Out"=w55:errorcluster)  [unwired: 6 in]
        n12 = Merge Errors(w37, w55) -> (w54:errorcluster)
      }
      frame "Free Image Memory" {
        w74 = FALSE  # Enable?
        n13 = call "Image Distruction.vi"("error in"=w96, "Images"=w95) -> ("error out"=w76:errorcluster)  [unwired: 9 out]
        n14 = Unbundle By Name(w75) -> ("Match and Edge.Edge"=w73:refnum<vi>, "Match and Edge.Target Data"=w85:refnum<vi>, "Matching Curves"=w84:refnum<vi>, "Tracking"=w83:refnum<vi>, "Focus"=w82:refnum<vi>, "Find Focus"=w81:refnum<vi>, "Set Target"=w80:refnum<vi>, "Link Stage & Camera"=w79:refnum<vi>, "Align"=w78:refnum<vi>)
        n15 = Build Array(w73, w85, w84, w83, w82, w81, w80, w79, w78) -> (w77:refnum<vi>[])
        n16 = call "Set Enable State on Multiple Controls.vi"("error in (no error)"=w76, "Enable?"=w74, "Controls"=w77) -> ("error out"=w67:errorcluster)  [unwired: 8 in]
        n17 = Unbundle By Name(w86) -> ("AutoFocus.Status"=w89:refnum<notifier>)
        n18 = Unbundle By Name(w75) -> ("Instrument Status"=w68:refnum<vi>)
        n19 = control-ref of="Instrument Status"() -> (w69:refnum<vi>)
        n20 = call "Notify.vi"("error in (no error)"=w67, "String"="Memory Deallocated", "Notifier in"=w89) -> ("error out"=w88:errorcluster)  [unwired: 8 in]
        n21 = call "Edit All Status Indicators.vi"("Instrument Status Ouside"=w68, "Instrument Status Inside"=w69, "Error In"=w67, "State"=Instrument_Status_State."Disconnected") -> ("Error Out"=w66:errorcluster)  [unwired: 6 in]
        n22 = Merge Errors(w88, w66) -> (w87:errorcluster)
      }
      frame "Set Match Criteria" {
        n23 = Unbundle By Name(w106) -> ("Instrument Status"=w99:refnum<vi>)
        n24 = control-ref of="Instrument Status"() -> (w98:refnum<vi>)
        n25 = call "Edit All Status Indicators.vi"("Instrument Status Ouside"=w99, "Instrument Status Inside"=w98, "Error In"=w108, "State"=Instrument_Status_State."Configuring") -> ("Error Out"=w107:errorcluster)  [unwired: 6 in]
        n26 = call "Target.vi"("error in (no error)"=w107, "Pattern Matching Criteria"="Matching Criteria", "Function"=Target_Functions."Setup Match Criteria") -> ("error out"=w110:errorcluster)  [unwired: 6 in, 2 out]
        n27 = Unbundle By Name(w105) -> ("AutoFocus.Status"=w113:refnum<notifier>)
        n28 = Unbundle By Name(w106) -> ("Instrument Status"=w102:refnum<vi>)
        n29 = control-ref of="Instrument Status"() -> (w101:refnum<vi>)
        n30 = call "Notify.vi"("error in (no error)"=w110, "String"="Match Criteria Updated", "Notifier in"=w113) -> ("error out"=w111:errorcluster)  [unwired: 8 in]
        n31 = call "Edit All Status Indicators.vi"("Instrument Status Ouside"=w102, "Instrument Status Inside"=w101, "Error In"=w110, "State"=Instrument_Status_State."Idle") -> ("Error Out"=w112:errorcluster)  [unwired: 6 in]
        n32 = Merge Errors(w111, w112) -> (w109:errorcluster)
      }
      frame "Set Target" {
        n33 = Unbundle By Name(w131) -> ("Instrument Status"=w127:refnum<vi>)
        n34 = control-ref of="Instrument Status"() -> (w126:refnum<vi>)
        n35 = call "Edit All Status Indicators.vi"("Instrument Status Ouside"=w127, "Instrument Status Inside"=w126, "Error In"=w143, "State"=Instrument_Status_State."Configuring") -> ("Error Out"=w140:errorcluster)  [unwired: 6 in]
        n36 = Unbundle By Name(w131) -> ("Match and Edge"=w149:T22)
        n37 = call "Target.vi"("Refnums"=w149, "Images"=w151, "error in (no error)"=w140, "Pattern Matching Criteria"=w150, "Function"=Target_Functions."Set Target") -> ("error out"=w152:errorcluster)  [unwired: 4 in, 2 out]
        n38 = call "Target.vi"("Refnums"=w149, "Images"=w151, "error in (no error)"=w152, "Pattern Matching Criteria"=w150, "Function"=Target_Functions."Find Target") -> ("error out"=w132:errorcluster, "Target Data"=w148:T5, "Target Found?"=w130:bool)  [unwired: 4 in]
        n39 = Unbundle By Name(w131) -> ("Matching Curves"=w139:refnum<vi>, "Tracking"=w138:refnum<vi>, "Focus"=w137:refnum<vi>, "Find Focus"=w136:refnum<vi>, "Link Stage & Camera"=w135:refnum<vi>, "Align"=w134:refnum<vi>)
        n40 = Build Array(w139, w138, w137, w136, w135, w134) -> (w133:refnum<vi>[])
        n41 = call "Set Enable State on Multiple Controls.vi"("error in (no error)"=w132, "Enable?"=w130, "Controls"=w133) -> ("error out"=w129:errorcluster)  [unwired: 8 in]
        n42 = Unbundle By Name(w141) -> ("AutoFocus.Status"=w144:refnum<notifier>)
        n43 = Unbundle By Name(w131) -> ("Instrument Status"=w123:refnum<vi>)
        n44 = control-ref of="Instrument Status"() -> (w122:refnum<vi>)
        n45 = call "Notify.vi"("error in (no error)"=w129, "String"="Target Set", "Notifier in"=w144) -> ("error out"=w146:errorcluster)  [unwired: 8 in]
        n46 = call "Edit All Status Indicators.vi"("Instrument Status Ouside"=w123, "Instrument Status Inside"=w122, "Error In"=w129, "State"=Instrument_Status_State."Idle") -> ("Error Out"=w145:errorcluster)  [unwired: 6 in]
        n47 = Merge Errors(w146, w145) -> (w142:errorcluster)
      }
      frame "Find Target" {
        n48 = Unbundle By Name(w171) -> ("Instrument Status"=w166:refnum<vi>)
        n49 = control-ref of="Instrument Status"() -> (w165:refnum<vi>)
        n50 = call "Edit All Status Indicators.vi"("Instrument Status Ouside"=w166, "Instrument Status Inside"=w165, "Error In"=w168, "State"=Instrument_Status_State."Measuring") -> ("Error Out"=w169:errorcluster)  [unwired: 6 in]
        n51 = Unbundle By Name(w171) -> ("Match and Edge.Image"=w178:refnum<vi>)
        n52 = call "Grab Frame.vi"("error in (no error)"=w169, "Image Refnum"=w178, "Images"=w180, "Notifiers"=w170) -> ("error out"=w179:errorcluster)  [unwired: 6 in, 1 out]
        n53 = Unbundle By Name(w171) -> ("Match and Edge"=w184:T22)
        n54 = call "Target.vi"("Refnums"=w184, "Images"=w180, "error in (no error)"=w179, "Pattern Matching Criteria"=w183, "Function"=Target_Functions."Find Target") -> ("error out"=w162:errorcluster, "Target Data"=w176:T5, "Target Found?"=w175:bool)  [unwired: 4 in]
        n55 = Unbundle By Name(w170) -> ("AutoFocus.Status"=w163:refnum<notifier>)
        n56 = Unbundle By Name(w171) -> ("Instrument Status"=w159:refnum<vi>)
        n57 = control-ref of="Instrument Status"() -> (w158:refnum<vi>)
        n58 = call "Notify.vi"("error in (no error)"=w162, "String"="Target Found", "Notifier in"=w163) -> ("error out"=w160:errorcluster)  [unwired: 8 in]
        n59 = call "Edit All Status Indicators.vi"("Instrument Status Ouside"=w159, "Instrument Status Inside"=w158, "Error In"=w162, "State"=Instrument_Status_State."Idle") -> ("Error Out"=w173:errorcluster)  [unwired: 6 in]
        n60 = Merge Errors(w160, w173) -> (w172:errorcluster)
      }
      frame "Grab Image" {
        w198 = TRUE  # Enable?
        n61 = Unbundle By Name(w194) -> ("Instrument Status"=w188:refnum<vi>)
        n62 = control-ref of="Instrument Status"() -> (w187:refnum<vi>)
        n63 = call "Edit All Status Indicators.vi"("Instrument Status Ouside"=w188, "Instrument Status Inside"=w187, "Error In"=w202, "State"=Instrument_Status_State."Measuring") -> ("Error Out"=w203:errorcluster)  [unwired: 6 in]
        n64 = Unbundle By Name(w194) -> ("Match and Edge.Image"=w209:refnum<vi>)
        n65 = call "Grab Frame.vi"("error in (no error)"=w203, "Image Refnum"=w209, "Images"=w210, "Notifiers"=w200) -> ("error out"=w197:errorcluster)  [unwired: 6 in, 1 out]
        n66 = Unbundle By Name(w194) -> ("Set Target"=w199:refnum<vi>)
        n67 = Build Array(w199) -> (w195:refnum<vi>[])
        n68 = call "Set Enable State on Multiple Controls.vi"("error in (no error)"=w197, "Enable?"=w198, "Controls"=w195) -> ("error out"=w196:errorcluster)  [unwired: 8 in]
        n69 = Unbundle By Name(w200) -> ("AutoFocus.Status"=w204:refnum<notifier>)
        n70 = Unbundle By Name(w194) -> ("Instrument Status"=w190:refnum<vi>)
        n71 = control-ref of="Instrument Status"() -> (w191:refnum<vi>)
        n72 = call "Notify.vi"("error in (no error)"=w196, "String"="Image Acquired", "Notifier in"=w204) -> ("error out"=w206:errorcluster)  [unwired: 8 in]
        n73 = call "Edit All Status Indicators.vi"("Instrument Status Ouside"=w190, "Instrument Status Inside"=w191, "Error In"=w196, "State"=Instrument_Status_State."Idle") -> ("Error Out"=w205:errorcluster)  [unwired: 6 in]
        n74 = Merge Errors(w206, w205) -> (w201:errorcluster)
      }
      frame "Get ROI" {
        n75 = Unbundle By Name(w216) -> ("Match and Edge.Image"=w219:refnum<vi>)
        n76 = property on="Property Node" class="ImageControl"(reference=w219, error in=w218) -> (error out=w217:errorcluster, "ROI"=w215:T34)  [unwired: 1 out]
      }
      frame "Set ROI" {
        n77 = Unbundle By Name(w228) -> ("Match and Edge.Image"=w231:refnum<vi>)
        n78 = property on="Property Node" class="ImageControl"(reference=w231, error in=w230, "ROI"=w227) -> (error out=w229:errorcluster)  [unwired: 1 out]
      }
      frame "Link Stage & Camera" {
        w264 = T29 {"Connection Settings"={"Tango VISA"="", "Baudrate"=57600, "Show Protocol?"=FALSE}, "Manual Control"={"North"=FALSE, "South"=FALSE, "West"=FALSE, "East"=FALSE, "Up"=FALSE, "Down"=FALSE, "Stop"=FALSE, "XY Step"=0.0, "Z step"=0.0}, "Coordinate Control"={"Motion Mode"=enum."Absolute", "Destination [mm]"=[]}} ("Configuration")
        n79 = Unbundle By Name(w253) -> ("Instrument Status"=w241:refnum<vi>)
        n80 = control-ref of="Instrument Status"() -> (w240:refnum<vi>)
        n81 = call "Edit All Status Indicators.vi"("Instrument Status Ouside"=w241, "Instrument Status Inside"=w240, "Error In"=w252, "State"=Instrument_Status_State."Configuring") -> ("Error Out"=w251:errorcluster)  [unwired: 6 in]
        n82 = Unbundle By Name(w254) -> ("XYZ Stage.Measurement"=w311:refnum<notifier>)
        n83 = Unbundle By Name(w269) -> ("XYZ Stage"=w309:refnum<queue>)
        n84 = Cancel Notification(0:w311, 3:w251) -> (8:w312:refnum<notifier>, 11:w238:errorcluster)  [unwired: 1 out]
        n85 = Wait on Notification(notifier=w312, error in (no error)=w238) -> (notification=w304:variant, error out=w310:errorcluster)  [unwired: 2 in, 2 out]
        n86 = call "Enqueue Message (Single).vi"("error in (no error)"=w238, "Message"="Get Status", "Message Queue"=w309) -> ("error out"=w307:errorcluster)  [unwired: 1 in, 7 out]
        n87 = Merge Errors(w307, w310) -> (w306:errorcluster)
        n88 = Multiply(x=dbl[] [1.0, 0.0, 0.0] ("PosOut"), y="Displacement") -> (x*y=w296:dbl[])
        n89 = Multiply(x=dbl[] [0.0, 1.0, 0.0] ("PosOut"), y="Displacement") -> (x*y=w295:dbl[])
        n90 = Variant To Data(error in=w306, type=dbl[] [] ("PosOut"), Variant=w304) -> (data=w297:dbl[], error out=w303:errorcluster)
        n91 = Add(x=w297, y=w295) -> (x+y=w298:dbl[])
        n92 = Add(x=w297, y=w296) -> (x+y=w299:dbl[])
        n93 = Bundle By Name(cluster=w264, "Coordinate Control.Destination [mm]"=w297) -> (w268:T29)
        n94 = Bundle By Name(cluster=w264, "Coordinate Control.Destination [mm]"=w299) -> (w301:T29)
        n95 = Bundle By Name(cluster=w264, "Coordinate Control.Destination [mm]"=w298) -> (w300:T29)
        n96 = Build Array(w268, w301, w300) -> (w302:T29[])
        n97 = for {
          tunnel: w261 -> [w321]
          tunnel: w313 -> [w340]
          tunnel: w253 -> [w322]
          tunnel: w269 -> [w332]
          shift-right: [w339] -> w271
          shift-left: w303 -> [w333]
          tunnel: w254 -> [w324]
          tunnel: w302 -> [w329] mode=indexing
          tunnel: [w327] -> w279 mode=indexing
          n98 = Unbundle By Name(w324) -> ("XYZ Stage.Status"=w334:refnum<notifier>)
          n99 = Cancel Notification(0:w334, 3:w333) -> (8:w330:refnum<notifier>, 11:w331:errorcluster)  [unwired: 1 out]
          n100 = Unbundle By Name(w332) -> ("XYZ Stage"=w336:refnum<queue>)
          n101 = Wait on Notification(notifier=w330, error in (no error)=w331) -> (error out=w335:errorcluster)  [unwired: 2 in, 3 out]
          n102 = Unbundle By Name(w322) -> ("Match and Edge.Image"=w323:refnum<vi>)
          n103 = call "Wait.vi"("error in (no error)"=w335, "milliseconds to wait"=u32 500) -> ("error out"=w320:errorcluster)  [unwired: 9 in]
          n104 = call "Enqueue Message (Single).vi"("error in (no error)"=w331, "Message Data"=w329, "Message"="Move", "Message Queue"=w336) -> ("error out"=w338:errorcluster)  [unwired: 7 out]
          n105 = Merge Errors(w338, w320) -> (w325:errorcluster)
          n106 = call "Grab Frame.vi"("error in (no error)"=w325, "Image Refnum"=w323, "Images"=w321, "Notifiers"=w324) -> ("error out"=w326:errorcluster)  [unwired: 6 in, 1 out]
          n107 = Unbundle By Name(w322) -> ("Match and Edge"=w342:T22)
          n108 = call "Target.vi"("Refnums"=w342, "Images"=w321, "error in (no error)"=w326, "Pattern Matching Criteria"=w340, "Function"=Target_Functions."Find Target") -> ("error out"=w339:errorcluster, "Target Data"=w328:T5)  [unwired: 4 in, 1 out]
          n109 = Unbundle By Name(w328) -> ("Match.Position"=w327:cluster{"x":sgl, "y":sgl})
        }
        n110 = Unbundle By Name(w254) -> ("XYZ Stage.Status"=w275:refnum<notifier>)
        n111 = Cancel Notification(0:w275, 3:w271) -> (8:w277:refnum<notifier>, 11:w276:errorcluster)  [unwired: 1 out]
        n112 = Unbundle By Name(w269) -> ("XYZ Stage"=w274:refnum<queue>)
        n113 = Wait on Notification(notifier=w277, error in (no error)=w276) -> (error out=w259:errorcluster)  [unwired: 2 in, 3 out]
        n114 = Index Array(array=w279, index #1=0 ("index"), index #2=1 ("index"), index #3=2 ("index")) -> (element #1=w283:cluster{"x":sgl, "y":sgl}, element #2=w284:cluster{"x":sgl, "y":sgl}, element #3=w285:cluster{"x":sgl, "y":sgl})
        n115 = call "Enqueue Message (Single).vi"("error in (no error)"=w276, "Message Data"=w268, "Message"="Move", "Message Queue"=w274) -> ("error out"=w272:errorcluster)  [unwired: 7 out]
        n116 = call "Wait.vi"("error in (no error)"=w259, "milliseconds to wait"=u32 500) -> ("error out"=w258:errorcluster)  [unwired: 9 in]
        n117 = Subtract(x=w284, y=w283) -> (x-y=w286:cluster{"x":sgl, "y":sgl})
        n118 = Subtract(x=w285, y=w283) -> (x-y=w287:cluster{"x":sgl, "y":sgl})
        n119 = Cluster To Array(cluster=w286) -> (array=w291:sgl[])
        n120 = Cluster To Array(cluster=w287) -> (array=w292:sgl[])
        n121 = Merge Errors(w272, w258) -> (w270:errorcluster)
        n122 = Build Array(w291, w292) -> (w288:sgl[][])
        n123 = Unbundle By Name(w253) -> ("Transformation Matrix"=w266:refnum<vi>)
        n124 = Divide(x=w288, y="Displacement") -> (x/y=w289:dbl[][])
        n125 = call-poly <vilib>:"Inverse Matrix.vi"("matrix type"=Matrix_Type_of_Inverse_Matrix."General", "Input Matrix"=w289) -> ("Inverse Matrix"=w265:T4)  [unwired: 1 out]
        n126 = Not A Number/Path/Refnum?(number/path/refnum=w266) -> (NaN/Path/Refnum?=w267:bool)
        n127 = case shown="False" w267 {
          tunnel: w270 -> [w317 w318]
          tunnel: [w316 w318] -> w263
          tunnel: w266 -> [w315 _]
          tunnel: w265 -> [w314 _]
          frame False {
            n128 = property class="Arr (strict)"(reference=w315, error in=w317, "Value"=w314) -> (error out=w316:errorcluster)  [unwired: 1 out]
          }
          frame True {
          }
        }
        n129 = Unbundle By Name(w253) -> ("Match and Edge.Image"=w262:refnum<vi>)
        n130 = call "Grab Frame.vi"("error in (no error)"=w263, "Image Refnum"=w262, "Images"=w261, "Notifiers"=w254) -> ("error out"=w247:errorcluster)  [unwired: 6 in, 1 out]
        n131 = Unbundle By Name(w253) -> ("Instrument Status"=w244:refnum<vi>)
        n132 = control-ref of="Instrument Status"() -> (w243:refnum<vi>)
        n133 = Unbundle By Name(w254) -> ("AutoFocus.Status"=w248:refnum<notifier>)
        n134 = call "Notify.vi"("error in (no error)"=w247, "String"="Stage and Camera Linked", "Notifier in"=w248) -> ("error out"=w245:errorcluster)  [unwired: 8 in]
        n135 = call "Edit All Status Indicators.vi"("Instrument Status Ouside"=w244, "Instrument Status Inside"=w243, "Error In"=w247, "State"=Instrument_Status_State."Idle") -> ("Error Out"=w255:errorcluster)  [unwired: 6 in]
        n136 = Merge Errors(w245, w255) -> (w250:errorcluster)
      }
      frame "Set Transformation Matrix" {
      }
      frame "Find Focus" {
        w369 = cluster{"Z (um)":dbl[], "Score":sgl[]} {"Z (um)"=[], "Score"=[]} ("Pattern Matching Focus Plot")
        # "Last value is complete array"
        n137 = Unbundle By Name(w370) -> ("Instrument Status"=w361:refnum<vi>)
        n138 = control-ref of="Instrument Status"() -> (w360:refnum<vi>)
        n139 = call "Edit All Status Indicators.vi"("Instrument Status Ouside"=w361, "Instrument Status Inside"=w360, "Error In"=w375, "State"=Instrument_Status_State."Moving") -> ("Error Out"=w374:errorcluster)  [unwired: 6 in]
        n140 = Unbundle By Name(w371) -> ("XYZ Stage.Measurement"=w400:refnum<notifier>)
        n141 = Unbundle By Name(w391) -> ("XYZ Stage"=w397:refnum<queue>)
        n142 = Cancel Notification(0:w400, 3:w374) -> (8:w401:refnum<notifier>, 11:w399:errorcluster)  [unwired: 1 out]
        n143 = call "Enqueue Message (Single).vi"("error in (no error)"=w374, "Message"="Get Status", "Message Queue"=w397) -> ("error out"=w395:errorcluster)  [unwired: 1 in, 7 out]
        n144 = Wait on Notification(notifier=w401, error in (no error)=w399) -> (notification=w392:variant, error out=w398:errorcluster)  [unwired: 2 in, 2 out]
        n145 = Merge Errors(w395, w398) -> (w394:errorcluster)
        n146 = Variant To Data(error in=w394, type=dbl[] [] ("PosOut"), Variant=w392) -> (data=w365:dbl[], error out=w389:errorcluster)
        n147 = call "ZScanRange.vi"("error in (no error)"=w389, "Z Scan Parameters"=w363) -> ("error out"=w388:errorcluster, "Displacements"=w368:dbl[])  [unwired: 7 in, 1 out]
        n148 = for {
          tunnel: w403 -> [w440]
          tunnel: w402 -> [w453]
          tunnel: w370 -> [w426]
          tunnel: w391 -> [w447]
          shift-right: [w424] -> w367
          shift-left: w388 -> [w448]
          tunnel: w371 -> [w441]
          shift-right: [w421] -> _
          shift-left: w369 -> [w422]
          shift-right: [w419] -> _
          shift-left: w369 -> [w420]
          tunnel: w368 -> [w411] mode=indexing
          tunnel: [w414] -> w366
          tunnel: w365 -> [w410]
          tunnel: [w405] -> w364
          w412 = 0.0
          # "Select Edge Analisys Score with Matching"
          # "Insert Edge Analisys Score to Array"
          # "Insert Pattern Matching Score to Array"
          n149 = Build Array(w412, w412, w411) -> (w409:dbl[])
          n150 = Add(x=w410, y=w409) -> (x+y=w407:dbl[])
          n151 = Bundle By Name(cluster=T29 {"Connection Settings"={"Tango VISA"="", "Baudrate"=57600, "Show Protocol?"=FALSE}, "Manual Control"={"North"=FALSE, "South"=FALSE, "West"=FALSE, "East"=FALSE, "Up"=FALSE, "Down"=FALSE, "Stop"=FALSE, "XY Step"=0.0, "Z step"=0.0}, "Coordinate Control"={"Motion Mode"=enum."Absolute", "Destination [mm]"=[]}} ("Configuration"), "Coordinate Control.Destination [mm]"=w407) -> (w406:T29)
          n152 = Unbundle By Name(w441) -> ("XYZ Stage.Status"=w449:refnum<notifier>)
          n153 = Unbundle By Name(w420) -> ("Z (um)"=w436:dbl[])
          n154 = Insert Into Array(array=w436, new element=w411) -> (w431:dbl[])  [unwired: 1 in]
          n155 = Cancel Notification(0:w449, 3:w448) -> (8:w445:refnum<notifier>, 11:w446:errorcluster)  [unwired: 1 out]
          n156 = Unbundle By Name(w447) -> ("XYZ Stage"=w450:refnum<queue>)
          n157 = Wait on Notification(notifier=w445, error in (no error)=w446) -> (error out=w438:errorcluster)  [unwired: 2 in, 3 out]
          n158 = call "Wait.vi"("error in (no error)"=w438, "milliseconds to wait"=u32 700) -> ("error out"=w437:errorcluster)  [unwired: 9 in]
          n159 = call "Enqueue Message (Single).vi"("error in (no error)"=w446, "Message Data"=w406, "Message"="Move", "Message Queue"=w450) -> ("error out"=w452:errorcluster)  [unwired: 7 out]
          n160 = Merge Errors(w452, w437) -> (w442:errorcluster)
          n161 = call "Grab Frame.vi"("error in (no error)"=w442, "Images"=w440, "Notifiers"=w441) -> ("error out"=w443:errorcluster)  [unwired: 7 in, 1 out]
          n162 = Unbundle By Name(w426) -> ("Match and Edge"=w455:T22)
          n163 = Unbundle By Name(w422) -> ("Score"=w435:sgl[])
          n164 = call "Target.vi"("Refnums"=w455, "Images"=w440, "error in (no error)"=w443, "Pattern Matching Criteria"=w453, "Function"=Target_Functions."Find Target") -> ("error out"=w425:errorcluster, "Target Data"=w444:T5)  [unwired: 4 in, 1 out]
          n165 = Unbundle By Name(w420) -> ("Score"=w433:sgl[])
          n166 = Unbundle By Name(w444) -> ("Match.Score"=w430:sgl, "Edge Analysis.Mean Value"=w429:sgl)
          n167 = Insert Into Array(array=w435, new element=w430) -> (w434:sgl[])  [unwired: 1 in]
          n168 = Bundle By Name(cluster=w422, "Z (um)"=w431, "Score"=w434) -> (w421:cluster{"Z (um)":dbl[], "Score":sgl[]})
          n169 = Insert Into Array(array=w433, new element=w429) -> (w432:sgl[])  [unwired: 1 in]
          n170 = call "Select Higher than Threshold.vi"("Function In"=w421) -> ("Function Out"=w418:cluster{"Z":dbl[], "Score":sgl[]}, "Indexes"=w423:i32[])
          n171 = Bundle By Name(cluster=w420, "Z (um)"=w431, "Score"=w432) -> (w419:cluster{"Z (um)":dbl[], "Score":sgl[]})
          n172 = Unbundle By Name(w426) -> ("Matching Curves"=w428:refnum<vi>)
          n173 = call "Select Index.vi"("Indexes"=w423, "Function In"=w419) -> ("Function Out"=w405:cluster{"Z":dbl[], "Score":sgl[]})  [unwired: 1 in, 2 out]
          n174 = call "Normalize.vi"("Focus Curve In"=w405) -> ("min"=w415:sgl, "Focus Curve Out"=w404:cluster{"Z (um)":dbl[], "Score":sgl[]}, "max"=w416:sgl)  [unwired: 2 in]
          n175 = Not A Number/Path/Refnum?(number/path/refnum=w428) -> (NaN/Path/Refnum?=w427:bool)
          n176 = Build Array(w418, w404) -> (w417:cluster{"Z (um)":dbl[], "Score":sgl[]}[])
          "Matching Curves" <- w417
          n177 = case shown="False" w427 {
            tunnel: w425 -> [w459 w460]
            tunnel: [w458 w460] -> w424
            tunnel: w428 -> [w457 _]
            tunnel: w417 -> [w456 _]
            frame False {
              n178 = property class="XYGraph (strict)"(reference=w457, error in=w459, "Value"=w456) -> (error out=w458:errorcluster)  [unwired: 1 out]
            }
            frame True {
            }
          }
          n179 = Bundle By Name(cluster=T1 {"Focus Plot"=[], "max"=0.0, "min"=0.0} ("output cluster"), "Focus Plot"=w417, "max"=w416, "min"=w415) -> (w414:T1)
        }
        n180 = call "Set Destination.vi"("Initial Position"=w365, "Scores with Matching"=w364) -> ("Configuration"=w380:T29)
        n181 = Unbundle By Name(w371) -> ("XYZ Stage.Status"=w384:refnum<notifier>)
        n182 = Cancel Notification(0:w384, 3:w367) -> (8:w386:refnum<notifier>, 11:w385:errorcluster)  [unwired: 1 out]
        n183 = Wait on Notification(notifier=w386, error in (no error)=w385) -> (error out=w378:errorcluster)  [unwired: 2 in, 3 out]
        n184 = Unbundle By Name(w391) -> ("XYZ Stage"=w383:refnum<queue>)
        n185 = call "Wait.vi"("error in (no error)"=w378, "milliseconds to wait"=u32 500) -> ("error out"=w377:errorcluster)  [unwired: 9 in]
        n186 = call "Enqueue Message (Single).vi"("error in (no error)"=w385, "Message Data"=w380, "Message"="Move", "Message Queue"=w383) -> ("error out"=w381:errorcluster)  [unwired: 7 out]
        n187 = Merge Errors(w381, w377) -> (w358:errorcluster)
        n188 = Unbundle By Name(w371) -> ("AutoFocus.Status"=w359:refnum<notifier>)
        n189 = Unbundle By Name(w370) -> ("Instrument Status"=w355:refnum<vi>)
        n190 = control-ref of="Instrument Status"() -> (w354:refnum<vi>)
        n191 = call "Edit All Status Indicators.vi"("Instrument Status Ouside"=w355, "Instrument Status Inside"=w354, "Error In"=w358, "State"=Instrument_Status_State."Idle") -> ("Error Out"=w373:errorcluster)  [unwired: 6 in]
        n192 = call "Notify.vi"("error in (no error)"=w358, "String"="Focus Corrected", "Notifier in"=w359) -> ("error out"=w356:errorcluster)  [unwired: 8 in]
        n193 = Merge Errors(w356, w373) -> (w372:errorcluster)
      }
      frame "Focus (Gradient)" {
        n194 = Unbundle By Name(w478) -> ("Instrument Status"=w477:refnum<vi>)
        n195 = control-ref of="Instrument Status"() -> (w476:refnum<vi>)
        n196 = call "Edit All Status Indicators.vi"("Instrument Status Ouside"=w477, "Instrument Status Inside"=w476, "Error In"=w481, "State"=Instrument_Status_State."Moving") -> ("Error Out"=w480:errorcluster)  [unwired: 6 in]
        n197 = Unbundle By Name(w486) -> ("XYZ Stage.Measurement"=w506:refnum<notifier>)
        n198 = Unbundle By Name(w485) -> ("XYZ Stage"=w504:refnum<queue>)
        n199 = Cancel Notification(0:w506, 3:w480) -> (8:w507:refnum<notifier>, 11:w490:errorcluster)  [unwired: 1 out]
        n200 = Wait on Notification(notifier=w507, error in (no error)=w490) -> (notification=w499:variant, error out=w505:errorcluster)  [unwired: 2 in, 2 out]
        n201 = call "Enqueue Message (Single).vi"("error in (no error)"=w490, "Message"="Get Status", "Message Queue"=w504) -> ("error out"=w502:errorcluster)  [unwired: 1 in, 7 out]
        n202 = Merge Errors(w502, w505) -> (w501:errorcluster)
        n203 = Variant To Data(error in=w501, type=dbl[] [] ("PosOut"), Variant=w499) -> (data=w470:dbl[], error out=w461:errorcluster)
        n204 = call "ZScanRange.vi"("error in (no error)"=w461, "Z Scan Parameters"=w469) -> ("error out"=w464:errorcluster, "Displacements"=w489:dbl[])  [unwired: 7 in, 1 out]
        n205 = Unbundle By Name(w469) -> ("Resolution"=w465:dbl, "Ascent Constant"=w468:dbl)
        n206 = Index Array(array=w470, index=2) -> (element=w466:dbl)
        n207 = call "Gradient Ascent.vi"("Function"=enum16{"Reset", "Ascend"}."Reset", "error in (no error)"=w464) -> ("error out"=w463:errorcluster)  [unwired: 11 in, 2 out]
        n208 = Subtract(x=w466, y=w465) -> (x-y=w467:dbl)
        n209 = for {
          tunnel: w509 -> [w556]
          tunnel: w508 -> [w564]
          tunnel: w478 -> [w523]
          shift-right: [w520] -> w492
          shift-left: w463 -> [w548]
          tunnel: w486 -> [w557]
          tunnel: w489 -> [w540] mode=indexing
          tunnel: w493 -> [w525]
          tunnel: w491 -> [w552]
          tunnel: [w543] -> w484
          tunnel: w487 -> [w549]
          tunnel: w486 -> [w546]
          tunnel: w485 -> [w545]
          shift-right: [w536] -> _
          shift-left: w470 -> [w528]
          tunnel: [w538] -> w472
          tunnel: w466 -> [w527]
          shift-right: [w535] -> _
          shift-left: w466 -> [w533]
          shift-left: w467 -> [w532]
          tunnel: w468 -> [w534]
          tunnel: w465 -> [w530]
          i -> [w543]
          stop <- w542 stop-if-true
          n210 = call "Grab Frame.vi"("error in (no error)"=w548, "Images"=w556, "Notifiers"=w557) -> ("error out"=w558:errorcluster)  [unwired: 7 in, 1 out]
          n211 = Unbundle By Name(w523) -> ("Match and Edge"=w566:T22)
          n212 = Subtract(x=w533, y=w532) -> (x-y=w531:dbl)
          n213 = call "Target.vi"("Refnums"=w566, "Images"=w556, "error in (no error)"=w558, "Pattern Matching Criteria"=w564, "Function"=Target_Functions."Find Target") -> ("error out"=w521:errorcluster, "Target Data"=w524:T5, "Target Found?"=w538:bool)  [unwired: 4 in]
          n214 = case shown="True" w538 {
            tunnel: w552 -> [_ w585]
            tunnel: w549 -> [_ w593]
            tunnel: w524 -> [_ w584]
            tunnel: w540 -> [w574 _]
            tunnel: [w575 w592] -> w539
            tunnel: [FALSE w590] -> w542
            tunnel: w533 -> [w572 w583]
            tunnel: w534 -> [_ w581]
            tunnel: w531 -> [_ w580]
            tunnel: w530 -> [_ w579]
            tunnel: w528 -> [w569 w578]
            tunnel: [w568 w578] -> w529
            tunnel: w527 -> [w567 _]
            frame False {
              n215 = call "Gradient Ascent.vi"("Function"=enum16{"Reset", "Ascend"}."Reset", "Z"=w572) -> ("Position Correction"=w576:dbl[])  [unwired: 11 in, 2 out]
              n216 = Replace Array Subset(array=w569, new element=w567, index=2) -> (w568:dbl[])
              n217 = Replace Array Subset(array=w576, new element=w574, index=2) -> (w575:dbl[])
            }
            frame True {
              n218 = call "Gradient Ascent.vi"("Function"=enum16{"Reset", "Ascend"}."Ascend", "Set Inverse Matrix"=w593, "Target Data"=w585, "Current Data"=w584, "Z"=w583, "Delta Z0"=w580, "Alpha"=w581) -> ("Position Correction"=w592:dbl[], "Delta Z"=w591:dbl)  [unwired: 6 in, 1 out]
              n219 = Multiply(x=w579, y=0.001) -> (x*y=w586:dbl)
              n220 = Absolute Value(x=w591) -> (abs(x)=w589:dbl)
              n221 = Absolute Value(x=w586) -> (abs(x)=w588:dbl)
              n222 = Less?(x=w589, y=w588) -> (x < y?=w590:bool)
            }
          }
          n223 = Add(x=w529, y=w539) -> (x+y=w536:dbl[])
          n224 = Index Array(array=w539, index=2) -> (element=w522:dbl)
          n225 = Unbundle By Name(w546) -> ("XYZ Stage.Status"=w561:refnum<notifier>)
          n226 = Bundle By Name(cluster=T29 {"Connection Settings"={"Tango VISA"="", "Baudrate"=57600, "Show Protocol?"=FALSE}, "Manual Control"={"North"=FALSE, "South"=FALSE, "West"=FALSE, "East"=FALSE, "Up"=FALSE, "Down"=FALSE, "Stop"=FALSE, "XY Step"=0.0, "Z step"=0.0}, "Coordinate Control"={"Motion Mode"=enum."Absolute", "Destination [mm]"=[]}} ("Configuration"), "Coordinate Control.Destination [mm]"=w536) -> (w550:T29)
          n227 = Cancel Notification(0:w561, 3:w521) -> (8:w559:refnum<notifier>, 11:w560:errorcluster)  [unwired: 1 out]
          n228 = Unbundle By Name(w545) -> ("XYZ Stage"=w547:refnum<queue>)
          n229 = call "Update Focus Chart.vi"("Refnums"=w523, "error in (no error)"=w521, "Current Z"=w522, "Target Data"=w524, "Focus Curve"=w525) -> ("error out"=w519:errorcluster, "Focus Plot"=w526:cluster{"Z (um)":dbl[], "Score":sgl[]}[])  [unwired: 5 in]
          n230 = Wait on Notification(notifier=w559, error in (no error)=w560) -> (error out=w554:errorcluster)  [unwired: 2 in, 3 out]
          n231 = property on="Matching Curves" class="XYGraph (strict)"("Value"=w526) -> ()  [unwired: 2 in, 2 out]
          n232 = call "Wait.vi"("error in (no error)"=w554, "milliseconds to wait"=u32 700) -> ("error out"=w553:errorcluster)  [unwired: 9 in]
          n233 = call "Enqueue Message (Single).vi"("error in (no error)"=w560, "Message Data"=w550, "Message"="Move", "Message Queue"=w547) -> ("error out"=w563:errorcluster)  [unwired: 7 out]
          n234 = Merge Errors(w563, w553) -> (w544:errorcluster)
          n235 = Merge Errors(w544, w519) -> (w520:errorcluster)
          n236 = Index Array "Extract Z"(array=w536, index=2) -> (element=w535:dbl)
        }
        n237 = Array Size(array=w489) -> (size(s)=w488:i32)
        n238 = Decrement(x=w488) -> (x-1=w483:i32)
        n239 = case shown="True" w472 {
          tunnel: w484 -> [_ w518]
          tunnel: w483 -> [_ w516]
          tunnel: ["Focus Failed" w511] -> w482
          frame False {
          }
          frame True {
            n240 = Divide(x=w516, y=2) -> (x/y=w517:dbl)
            n241 = Greater?(x=w518, y=w517) -> (0:w514:bool)
            n242 = Select(t="Focus Corrected (Change Direction)", s=w514, f="Focus Corrected (Same Direction)") -> (s? t:f=w511:string)
          }
        }
        n243 = Unbundle By Name(w486) -> ("AutoFocus.Status"=w495:refnum<notifier>)
        n244 = Unbundle By Name(w478) -> ("Instrument Status"=w475:refnum<vi>)
        n245 = control-ref of="Instrument Status"() -> (w474:refnum<vi>)
        n246 = call "Notify.vi"("error in (no error)"=w492, "String"=w482, "Notifier in"=w495) -> ("error out"=w497:errorcluster)  [unwired: 8 in]
        n247 = call "Edit All Status Indicators.vi"("Instrument Status Ouside"=w475, "Instrument Status Inside"=w474, "Error In"=w492, "State"=Instrument_Status_State."Idle") -> ("Error Out"=w496:errorcluster)  [unwired: 6 in]
        n248 = Merge Errors(w497, w496) -> (w494:errorcluster)
      }
      frame "Focus (Threshold)" {
        n249 = Unbundle By Name(w602) -> ("Instrument Status"=w615:refnum<vi>)
        n250 = control-ref of="Instrument Status"() -> (w614:refnum<vi>)
        n251 = call "Edit All Status Indicators.vi"("Instrument Status Ouside"=w615, "Instrument Status Inside"=w614, "Error In"=w618, "State"=Instrument_Status_State."Moving") -> ("Error Out"=w617:errorcluster)  [unwired: 6 in]
        n252 = Unbundle By Name(w600) -> ("XYZ Stage.Measurement"=w636:refnum<notifier>)
        n253 = Unbundle By Name(w603) -> ("XYZ Stage"=w634:refnum<queue>)
        n254 = Cancel Notification(0:w636, 3:w617) -> (8:w637:refnum<notifier>, 11:w622:errorcluster)  [unwired: 1 out]
        n255 = Wait on Notification(notifier=w637, error in (no error)=w622) -> (notification=w629:variant, error out=w635:errorcluster)  [unwired: 2 in, 2 out]
        n256 = call "Enqueue Message (Single).vi"("error in (no error)"=w622, "Message"="Get Status", "Message Queue"=w634) -> ("error out"=w632:errorcluster)  [unwired: 1 in, 7 out]
        n257 = Merge Errors(w632, w635) -> (w631:errorcluster)
        n258 = Variant To Data(error in=w631, type=dbl[] [] ("PosOut"), Variant=w629) -> (data=w595:dbl[], error out=w628:errorcluster)
        n259 = call "ZScanRange.vi"("error in (no error)"=w628, "Z Scan Parameters"=w607) -> ("error out"=w609:errorcluster, "Displacements"=w608:dbl[])  [unwired: 7 in, 1 out]
        n260 = Index Array(array=w595, index=2) -> (element=w596:dbl)
        n261 = for {
          tunnel: w601 -> [w672]
          tunnel: w599 -> [w680]
          tunnel: w602 -> [w651]
          shift-right: [w652] -> w606
          shift-left: w609 -> [w663]
          tunnel: w600 -> [w673]
          tunnel: w608 -> [w647] mode=indexing
          tunnel: w598 -> [w646]
          tunnel: [w664] -> w605
          tunnel: w604 -> [w643]
          tunnel: w600 -> [w660]
          tunnel: w603 -> [w659]
          shift-right: [w638] -> _
          shift-left: w595 -> [w662]
          tunnel: w596 -> [w654]
          tunnel: w607 -> [w657]
          tunnel: [w644] -> w597
          tunnel: w594 -> [w649]
          i -> [w664]
          stop <- w668 stop-if-true
          w639 = 0.0 ("element")
          # "Stop if Matching \nHigher than Threshold"
          n262 = call "Grab Frame.vi"("error in (no error)"=w663, "Images"=w672, "Notifiers"=w673) -> ("error out"=w674:errorcluster)  [unwired: 7 in, 1 out]
          n263 = Unbundle By Name(w651) -> ("Match and Edge"=w682:T22)
          n264 = Replace Array Subset(array=w662, new element=w654, index=2) -> (w642:dbl[])
          n265 = call "Target.vi"("Refnums"=w682, "Images"=w672, "error in (no error)"=w674, "Pattern Matching Criteria"=w680, "Function"=Target_Functions."Find Target") -> ("error out"=w648:errorcluster, "Target Data"=w645:T5, "Target Found?"=w644:bool)  [unwired: 4 in]
          n266 = Unbundle By Name(w657) -> ("Focus Threshold"=w656:dbl)
          n267 = Unbundle By Name(w645) -> ("Match.Score"=w667:sgl)
          n268 = Greater?(x=w667, y=w656) -> (0:w668:bool)
          n269 = call "CompensateXY.vi"("Inverse Matrix"=w643, "Current Data"=w645, "Target Found?"=w644, "Target Data"=w646) -> ("XY Displacement"=w641:dbl[])
          n270 = Build Array(w639, w639, w647) -> (w640:dbl[])
          n271 = Compound Arithmetic op=ADD(w642, w641, w640) -> (w638:dbl[])
          n272 = Unbundle By Name(w660) -> ("XYZ Stage.Status"=w677:refnum<notifier>)
          n273 = Bundle By Name(cluster=T29 {"Connection Settings"={"Tango VISA"="", "Baudrate"=57600, "Show Protocol?"=FALSE}, "Manual Control"={"North"=FALSE, "South"=FALSE, "West"=FALSE, "East"=FALSE, "Up"=FALSE, "Down"=FALSE, "Stop"=FALSE, "XY Step"=0.0, "Z step"=0.0}, "Coordinate Control"={"Motion Mode"=enum."Absolute", "Destination [mm]"=[]}} ("Configuration"), "Coordinate Control.Destination [mm]"=w638) -> (w665:T29)
          n274 = Cancel Notification(0:w677, 3:w648) -> (8:w675:refnum<notifier>, 11:w676:errorcluster)  [unwired: 1 out]
          n275 = call "Update Focus Chart.vi"("Refnums"=w651, "error in (no error)"=w648, "Current Z"=w647, "Target Data"=w645, "Focus Curve"=w649) -> ("error out"=w650:errorcluster, "Focus Plot"=w653:cluster{"Z (um)":dbl[], "Score":sgl[]}[])  [unwired: 5 in]
          n276 = Unbundle By Name(w659) -> ("XYZ Stage"=w661:refnum<queue>)
          n277 = property on="Matching Curves" class="XYGraph (strict)"("Value"=w653) -> ()  [unwired: 2 in, 2 out]
          n278 = Wait on Notification(notifier=w675, error in (no error)=w676) -> (error out=w670:errorcluster)  [unwired: 2 in, 3 out]
          n279 = call "Wait.vi"("error in (no error)"=w670, "milliseconds to wait"=u32 700) -> ("error out"=w669:errorcluster)  [unwired: 9 in]
          n280 = call "Enqueue Message (Single).vi"("error in (no error)"=w676, "Message Data"=w665, "Message"="Move", "Message Queue"=w661) -> ("error out"=w679:errorcluster)  [unwired: 7 out]
          n281 = Merge Errors(w679, w669) -> (w658:errorcluster)
          n282 = Merge Errors(w658, w650) -> (w652:errorcluster)
        }
        n283 = Array Size(array=w608) -> (size(s)=w621:i32)
        n284 = Decrement(x=w621) -> (x-1=w620:i32)
        n285 = case shown="False" w597 {
          tunnel: w605 -> [_ w691]
          tunnel: w620 -> [_ w689]
          tunnel: ["Focus Failed" w684] -> w619
          frame False {
          }
          frame True {
            n286 = Divide(x=w689, y=2) -> (x/y=w690:dbl)
            n287 = Greater?(x=w691, y=w690) -> (0:w687:bool)
            n288 = Select(t="Focus Corrected (Change Direction)", s=w687, f="Focus Corrected (Same Direction)") -> (s? t:f=w684:string)
          }
        }
        n289 = Unbundle By Name(w600) -> ("AutoFocus.Status"=w624:refnum<notifier>)
        n290 = Unbundle By Name(w602) -> ("Instrument Status"=w613:refnum<vi>)
        n291 = control-ref of="Instrument Status"() -> (w612:refnum<vi>)
        n292 = call "Notify.vi"("error in (no error)"=w606, "String"=w619, "Notifier in"=w624) -> ("error out"=w626:errorcluster)  [unwired: 8 in]
        n293 = call "Edit All Status Indicators.vi"("Instrument Status Ouside"=w613, "Instrument Status Inside"=w612, "Error In"=w606, "State"=Instrument_Status_State."Idle") -> ("Error Out"=w625:errorcluster)  [unwired: 6 in]
        n294 = Merge Errors(w626, w625) -> (w623:errorcluster)
      }
      frame "Focus (Turning Points)" {
        n295 = Unbundle By Name(w717) -> ("Instrument Status"=w725:refnum<vi>)
        n296 = control-ref of="Instrument Status"() -> (w724:refnum<vi>)
        n297 = call "Edit All Status Indicators.vi"("Instrument Status Ouside"=w725, "Instrument Status Inside"=w724, "Error In"=w728, "State"=Instrument_Status_State."Moving") -> ("Error Out"=w727:errorcluster)  [unwired: 6 in]
        n298 = Unbundle By Name(w702) -> ("XYZ Stage.Measurement"=w743:refnum<notifier>)
        n299 = Unbundle By Name(w699) -> ("XYZ Stage"=w741:refnum<queue>)
        n300 = Cancel Notification(0:w743, 3:w727) -> (8:w744:refnum<notifier>, 11:w730:errorcluster)  [unwired: 1 out]
        n301 = Wait on Notification(notifier=w744, error in (no error)=w730) -> (notification=w736:variant, error out=w742:errorcluster)  [unwired: 2 in, 2 out]
        n302 = call "Enqueue Message (Single).vi"("error in (no error)"=w730, "Message"="Get Status", "Message Queue"=w741) -> ("error out"=w739:errorcluster)  [unwired: 1 in, 7 out]
        n303 = Merge Errors(w739, w742) -> (w738:errorcluster)
        n304 = Variant To Data(error in=w738, type=dbl[] [] ("PosOut"), Variant=w736) -> (data=w712:dbl[], error out=w708:errorcluster)
        n305 = call "AskTurning.vi"("error in (no error)"=w708, "Function"=enum16{"Turning?", "Reset"}."Reset") -> ("error out"=w707:errorcluster)  [unwired: 6 in, 3 out]
        n306 = call "ZScanRange.vi"("error in (no error)"=w708, "Z Scan Parameters"=w692) -> ("error out"=w719:errorcluster, "Displacements"=w705:dbl[], "Inspect?"=w706:bool[])  [unwired: 7 in]
        n307 = Merge Errors(w719, w707) -> (w709:errorcluster)
        n308 = Index Array(array=w712, index=2) -> (element=w713:dbl)
        n309 = for {
          tunnel: w716 -> [w809]
          tunnel: w715 -> [w811]
          tunnel: w717 -> [w802]
          shift-right: [w803] -> w703
          shift-left: w709 -> [w808]
          tunnel: w702 -> [w810]
          tunnel: w705 -> [w797] mode=indexing
          tunnel: w714 -> [w799]
          tunnel: w718 -> [w800]
          tunnel: w702 -> [w806]
          tunnel: w699 -> [w805]
          shift-right: [w796] -> w701
          shift-left: w712 -> [w807]
          tunnel: w713 -> [w804]
          tunnel: w711 -> [w801]
          shift-right: [w795] -> _
          shift-left: w706 -> [w793]
          tunnel: w705 -> [w792]
          shift-right: [w788] -> w695
          shift-left: _ -> [w787]
          shift-right: [w798] -> w697
          shift-left: FALSE ("Target Found?") -> [w791]
          shift-right: [w790] -> w700
          shift-left: _ -> [w789]
          tunnel: [w785] -> w696
          tunnel: w692 -> [w784]
          i -> [w786]
          n310 = Index Array(array=w793, index=w786) -> (element=w794:bool)
          n311 = case shown="True" w794 {
            tunnel: w811 -> [_ w867]
            tunnel: w810 -> [_ w865]
            tunnel: w809 -> [_ w864]
            tunnel: w808 -> [w818 w836]
            tunnel: w807 -> [w817 w834]
            tunnel: w806 -> [_ w863]
            tunnel: w805 -> [_ w862]
            tunnel: w804 -> [w812 w823]
            tunnel: [w818 w828] -> w803
            tunnel: w802 -> [_ w860]
            tunnel: w801 -> [_ w859]
            tunnel: w800 -> [_ w858]
            tunnel: w799 -> [_ w857]
            tunnel: [w814 w822] -> w798
            tunnel: w797 -> [_ w832]
            tunnel: [w817 w852] -> w796
            tunnel: w793 -> [w816 w850]
            tunnel: [w816 w849] -> w795
            tunnel: w792 -> [_ w820]
            tunnel: [w815 w825] -> w788
            tunnel: w787 -> [w815 _]
            tunnel: w791 -> [w814 _]
            tunnel: [w813 w821] -> w790
            tunnel: w789 -> [w813 _]
            tunnel: w786 -> [_ w824]
            tunnel: [w812 w823] -> w785
            tunnel: w784 -> [_ w819]
            frame False {
            }
            frame True {
              w833 = 0.0 ("element")
              n312 = Unbundle By Name(w863) -> ("XYZ Stage.Status"=w846:refnum<notifier>)
              n313 = Build Array(w833, w833, w832) -> (w831:dbl[])
              n314 = Compound Arithmetic op=ADD(w834, w831) -> (w826:dbl[])
              n315 = Bundle By Name(cluster=T29 {"Connection Settings"={"Tango VISA"="", "Baudrate"=57600, "Show Protocol?"=FALSE}, "Manual Control"={"North"=FALSE, "South"=FALSE, "West"=FALSE, "East"=FALSE, "Up"=FALSE, "Down"=FALSE, "Stop"=FALSE, "XY Step"=0.0, "Z step"=0.0}, "Coordinate Control"={"Motion Mode"=enum."Absolute", "Destination [mm]"=[]}} ("Configuration"), "Coordinate Control.Destination [mm]"=w826) -> (w839:T29)
              n316 = Cancel Notification(0:w846, 3:w836) -> (8:w844:refnum<notifier>, 11:w845:errorcluster)  [unwired: 1 out]
              n317 = Unbundle By Name(w862) -> ("XYZ Stage"=w838:refnum<queue>)
              n318 = Wait on Notification(notifier=w844, error in (no error)=w845) -> (error out=w842:errorcluster)  [unwired: 2 in, 3 out]
              n319 = call "Wait.vi"("error in (no error)"=w842, "milliseconds to wait"=u32 700) -> ("error out"=w841:errorcluster)  [unwired: 9 in]
              n320 = call "Enqueue Message (Single).vi"("error in (no error)"=w845, "Message Data"=w839, "Message"="Move", "Message Queue"=w838) -> ("error out"=w848:errorcluster)  [unwired: 7 out]
              n321 = Merge Errors(w848, w841) -> (w835:errorcluster)
              n322 = call "Grab Frame.vi"("error in (no error)"=w835, "Images"=w864, "Notifiers"=w865) -> ("error out"=w866:errorcluster)  [unwired: 7 in, 1 out]
              n323 = Unbundle By Name(w860) -> ("Match and Edge"=w869:T22)
              n324 = Replace Array Subset(array=w826, new element=w823, index=2) -> (w856:dbl[])
              n325 = call "Target.vi"("Refnums"=w869, "Images"=w864, "error in (no error)"=w866, "Pattern Matching Criteria"=w867, "Function"=Target_Functions."Find Target") -> ("error out"=w829:errorcluster, "Target Data"=w854:T5, "Target Found?"=w822:bool)  [unwired: 4 in]
              n326 = call "CompensateXY.vi"("Inverse Matrix"=w858, "Current Data"=w854, "Target Found?"=w822, "Target Data"=w857) -> ("XY Displacement"=w855:dbl[])
              n327 = Unbundle By Name(w854) -> ("Edge Analysis.Mean Value"=w851:sgl)
              n328 = Compound Arithmetic op=ADD(w856, w855) -> (w852:dbl[])
              n329 = call "Update Focus Chart.vi"("Refnums"=w860, "error in (no error)"=w829, "Current Z"=w832, "Target Data"=w854, "Focus Curve"=w859) -> ("error out"=w830:errorcluster, "Focus Plot"=w837:cluster{"Z (um)":dbl[], "Score":sgl[]}[])  [unwired: 5 in]
              n330 = call "AskTurning.vi"("Z Scan Parameters"=w819, "error in (no error)"=w829, "Edge Sherpness"=w851, "Z"=w832, "Function"=enum16{"Turning?", "Reset"}."Turning?") -> ("error out"=w827:errorcluster, "Z @ Max Sharpness"=w821:dbl, "Questions"=w825:T35)  [unwired: 3 in, 1 out]
              n331 = property on="Matching Curves" class="XYGraph (strict)"("Value"=w837) -> ()  [unwired: 2 in, 2 out]
              n332 = call "UpdateInspect.vi"("Current Id"=w824, "Answers"=w825, "Current Z"=w832, "Displacements"=w820, "Inspect? in"=w850) -> ("Inspect? out"=w849:bool[])  [unwired: 6 in]
              n333 = Merge Errors(w827, w830) -> (w828:errorcluster)
            }
          }
        }
        n334 = Unbundle By Name(w695) -> ("Focus at Edge?"=w694:bool)
        n335 = case shown="True" w697 {
          selector: w697 -> [w745 _]
          tunnel: ["Focus Failed" w750] -> w729
          tunnel: [w746 w757] -> w704
          tunnel: w703 -> [w746 w756]
          tunnel: w702 -> [_ w755]
          tunnel: w701 -> [_ w752]
          tunnel: w700 -> [_ w754]
          tunnel: w699 -> [_ w753]
          tunnel: w696 -> [_ w751]
          tunnel: w694 -> [_ w748]
          tunnel: [w745 w749] -> w693
          frame False {
          }
          frame True {
            n336 = case shown="True" w748 {
              tunnel: [w770 w783] -> w757
              tunnel: w756 -> [w769 w783]
              tunnel: w755 -> [w768 _]
              tunnel: w754 -> [w764 _]
              tunnel: w753 -> [w763 _]
              tunnel: w752 -> [w761 _]
              tunnel: w751 -> [w760 _]
              tunnel: ["Focus Corrected" "Focus at Edge"] -> w750
              frame False {
                w766 = 0.0 ("element")
                n337 = Unbundle By Name(w768) -> ("XYZ Stage.Status"=w779:refnum<notifier>)
                n338 = Replace Array Subset(array=w761, new element=w760, index=2) -> (w759:dbl[])
                n339 = Build Array(w766, w766, w764) -> (w767:dbl[])
                n340 = Compound Arithmetic op=ADD(w759, w767) -> (w765:dbl[])
                n341 = Bundle By Name(cluster=T29 {"Connection Settings"={"Tango VISA"="", "Baudrate"=57600, "Show Protocol?"=FALSE}, "Manual Control"={"North"=FALSE, "South"=FALSE, "West"=FALSE, "East"=FALSE, "Up"=FALSE, "Down"=FALSE, "Stop"=FALSE, "XY Step"=0.0, "Z step"=0.0}, "Coordinate Control"={"Motion Mode"=enum."Absolute", "Destination [mm]"=[]}} ("Configuration"), "Coordinate Control.Destination [mm]"=w765) -> (w772:T29)
                n342 = Cancel Notification(0:w779, 3:w769) -> (8:w777:refnum<notifier>, 11:w778:errorcluster)  [unwired: 1 out]
                n343 = Unbundle By Name(w763) -> ("XYZ Stage"=w771:refnum<queue>)
                n344 = Wait on Notification(notifier=w777, error in (no error)=w778) -> (error out=w775:errorcluster)  [unwired: 2 in, 3 out]
                n345 = call "Wait.vi"("error in (no error)"=w775, "milliseconds to wait"=u32 500) -> ("error out"=w774:errorcluster)  [unwired: 9 in]
                n346 = call "Enqueue Message (Single).vi"("error in (no error)"=w778, "Message Data"=w772, "Message"="Move", "Message Queue"=w771) -> ("error out"=w781:errorcluster)  [unwired: 7 out]
                n347 = Merge Errors(w781, w774) -> (w770:errorcluster)
              }
              frame True {
              }
            }
            n348 = Not(x=w748) -> (.not. x?=w749:bool)
          }
        }
        n349 = Unbundle By Name(w702) -> ("AutoFocus.Status"=w732:refnum<notifier>)
        n350 = Unbundle By Name(w717) -> ("Instrument Status"=w723:refnum<vi>)
        n351 = control-ref of="Instrument Status"() -> (w722:refnum<vi>)
        n352 = call "Notify.vi"("error in (no error)"=w704, "String"=w729, "Notifier in"=w732) -> ("error out"=w734:errorcluster)  [unwired: 8 in]
        n353 = call "Edit All Status Indicators.vi"("Instrument Status Ouside"=w723, "Instrument Status Inside"=w722, "Error In"=w704, "State"=Instrument_Status_State."Idle") -> ("Error Out"=w733:errorcluster)  [unwired: 6 in]
        n354 = Merge Errors(w734, w733) -> (w731:errorcluster)
      }
      frame "Align" {
        n355 = Unbundle By Name(w883) -> ("Instrument Status"=w872:refnum<vi>)
        n356 = control-ref of="Instrument Status"() -> (w871:refnum<vi>)
        n357 = call "Edit All Status Indicators.vi"("Instrument Status Ouside"=w872, "Instrument Status Inside"=w871, "Error In"=w884, "State"=Instrument_Status_State."Moving") -> ()  [unwired: 6 in, 1 out]
        n358 = Unbundle By Name(w883) -> ("Match and Edge.Image"=w889:refnum<vi>)
        n359 = call "Grab Frame.vi"("error in (no error)"=w884, "Image Refnum"=w889, "Images"=w891, "Notifiers"=w885) -> ("error out"=w893:errorcluster)  [unwired: 6 in, 1 out]
        n360 = Unbundle By Name(w883) -> ("Match and Edge"=w895:T22)
        n361 = call "Target.vi"("Refnums"=w895, "Images"=w891, "error in (no error)"=w893, "Pattern Matching Criteria"=w898, "Function"=Target_Functions."Find Target") -> ("error out"=w897:errorcluster, "Target Data"=w880:T5, "Target Found?"=w881:bool)  [unwired: 4 in]
        n362 = case shown="True" w881 {
          tunnel: w897 -> [w899 w922]
          tunnel: [w899 w921] -> w877
          tunnel: w896 -> [_ w920]
          tunnel: w880 -> [_ w919]
          tunnel: w885 -> [_ w918]
          tunnel: w892 -> [_ w917]
          tunnel: w890 -> [_ w912]
          frame False {
          }
          frame True {
            n363 = Unbundle By Name(w919) -> ("Match.Position"=w903:cluster{"x":sgl, "y":sgl})
            n364 = Unbundle By Name(w912) -> ("Match.Position"=w904:cluster{"x":sgl, "y":sgl})
            n365 = Subtract(x=w904, y=w903) -> (x-y=w913:cluster{"x":sgl, "y":sgl})
            n366 = Cluster To Array(cluster=w913) -> (array=w916:sgl[])
            n367 = call-poly <vilib>:"A x B.vi"("Vector"=w916, "A"=w917) -> ("A x Vector"=w909:dbl[])  [unwired: 1 out]
            n368 = Index Array(array=w909, index #1=0 ("index"), index #2=1 ("index")) -> (element #1=w908:dbl, element #2=w907:dbl)
            n369 = Build Array(w908, w907, 0.0 ("element")) -> (w905:dbl[])
            n370 = Unbundle By Name(w918) -> ("XYZ Stage.Status"=w926:refnum<notifier>)
            n371 = Bundle By Name(cluster=T29 {"Connection Settings"={"Tango VISA"="", "Baudrate"=57600, "Show Protocol?"=FALSE}, "Manual Control"={"North"=FALSE, "South"=FALSE, "West"=FALSE, "East"=FALSE, "Up"=FALSE, "Down"=FALSE, "Stop"=FALSE, "XY Step"=0.0, "Z step"=0.0}, "Coordinate Control"={"Motion Mode"=enum."Relative", "Destination [mm]"=[]}} ("Configuration"), "Coordinate Control.Destination [mm]"=w905) -> (w915:T29)
            n372 = Cancel Notification(0:w926, 3:w922) -> (8:w928:refnum<notifier>, 11:w927:errorcluster)  [unwired: 1 out]
            n373 = Unbundle By Name(w920) -> ("XYZ Stage"=w925:refnum<queue>)
            n374 = Wait on Notification(notifier=w928, error in (no error)=w927) -> (error out=w901:errorcluster)  [unwired: 2 in, 3 out]
            n375 = call "Enqueue Message (Single).vi"("error in (no error)"=w927, "Message Data"=w915, "Message"="Move", "Message Queue"=w925) -> ("error out"=w923:errorcluster)  [unwired: 7 out]
            n376 = call "Wait.vi"("error in (no error)"=w901, "milliseconds to wait"=u32 500) -> ("error out"=w900:errorcluster)  [unwired: 9 in]
            n377 = Merge Errors(w923, w900) -> (w921:errorcluster)
          }
        }
        n378 = Unbundle By Name(w885) -> ("AutoFocus.Status"=w879:refnum<notifier>)
        n379 = Unbundle By Name(w883) -> ("Instrument Status"=w875:refnum<vi>)
        n380 = control-ref of="Instrument Status"() -> (w874:refnum<vi>)
        n381 = call "Notify.vi"("error in (no error)"=w877, "String"="Target Aligned", "Notifier in"=w879) -> ("error out"=w876:errorcluster)  [unwired: 8 in]
        n382 = call "Edit All Status Indicators.vi"("Instrument Status Ouside"=w875, "Instrument Status Inside"=w874, "Error In"=w877, "State"=Instrument_Status_State."Idle") -> ("Error Out"=w887:errorcluster)  [unwired: 6 in]
        n383 = Merge Errors(w876, w887) -> (w886:errorcluster)
      }
      frame "Update Refnums" {
        n384 = Unbundle By Name("Notifiers") -> ("AutoFocus.Status"=w931:refnum<notifier>)
        n385 = call "Notify.vi"("error in (no error)"=w930, "String"="Refnums Updated", "Notifier in"=w931) -> ("error out"=w929:errorcluster)  [unwired: 8 in]
      }
    }
  }
  "error out" <- w6
  "Transformation Matrix" <- w5
  "Target Found?" <- w3
  "Target Data" <- w4
  "Edge Detection Array" <- w1
